vi "STED Control V6.vi"() -> ()   [LabVIEW 2014]
uses:
  FPGA-7842R-Reference.ctl
  Scan Parameters.ctl
  Manual Controls V2.ctl
  <vilib>/Utility/miscctls.llb/LVRectTypeDef.ctl
  Laser Controls.ctl
  Controls/StageStates.ctl
  <vilib>/Utility/miscctls.llb/LVPositionTypeDef.ctl
  Type Defs/Image Acquisition Parameters.ctl
  Detectors.ctl
  Type Defs/P541.ctl
  Tools VIs/GrpahTools.ctl
  Type Defs/N664.ctl
  Type Defs/M227.ctl
  Type Defs/P612.ctl
  Type Defs/M686.ctl
  Type Defs/P841.ctl
  Type Defs/ASI.ctl
  Type Defs/Image Control.ctl
panel:
  in  "Load Positions":bool
  in  "ASI":bool
  in  "4Pi Cavity Translation Z - ASI":T1={"Up ASI"=FALSE, "Down ASI"=FALSE, "Step Size (um)"=0.001, "Z (um)"=0.001, "F (um)"=0.001, "Velocity"=0.001} caption="ASI" {"Velocity" min=0.001; "F (um)" min=0.001; "Z (um)" min=0.001; "Step Size (um)" min=0.001}
  in  "Lower Shutter":bool
  in  "Upper Shutter":bool
  in  "Phase Compensation Mirror - P841 (0~15 um)":T2
  in  "Sample Stage XY - M686":T3 {"Y" format="%#_4g"; "X" format="%#_4g"}
  in  "Joystick Velocity":string(combo)
  in  "Radio Buttons":enum32{"Radio Selection 1", "Radio Selection 2"}(radio)
  in  "Bottom Objective Holder XY - P612 (0~100 um)":T4 {"Y" format="%#_4g"; "X" format="%#_4g"}
  in  "Upper Objective Holder Z - N664 (8~19 mm)":T5 {"Position" min=8.0 max=20.0 scale=8.0..20.0; "Step Size (um)" min=0.001}
  in  "Abort AllStage":bool
  in  "Stages":T6={"M227"=TRUE, "N664"=TRUE, "P612"=TRUE, "M686"=TRUE, "P841"=TRUE, "ASI"=TRUE}
  in  "Micrometer Sample Stage Holder Z - M227":T7
  in  "Cursor":bool
  in  "Graph Mode":T8=enum."FullChip"
  in  "Colormap":T9(ring)
  in  "Active Channel":u16(ring) items=["Channel 1"]
  in  "Graph Tools":T10
  in  "Tab Control":T11(tab)
  in  "SLM":bool
  in  "DM":bool
  in  "Timing":bool
  in  "Focus Control":T12
  out "Channel 6":sgl[][](graph)
  out "Channel 5":sgl[][](graph)
  out "Channel 4":sgl[][](graph)
  out "Channel 3":sgl[][](graph)
  out "Channel 2":sgl[][](graph)
  in  "Detectors":T13
  in  "Laser Controls":T14 {"STED Power (V)" scale=0.0..10.0}
  in  "Save File Path":path=path "C:/Users/ED STED/Desktop/temp.DBL"
  in  "Capture":bool
  out "Channel 1":sgl[][](graph)
  in  "Image Acquisition Parameters":T15={"Scan Type"=enum."Beam Scanning", "Scan Mode"=enum."XY", "Fast Axis Frequency (Hz)"=15780.0, "Image Format"=256, "Line Accumulations"=100, "Frames Per Capture"=1, "Frames Accumulations"=1, "Image Dimension (um)"=[15.0, 15.0], "Number of Z Steps"=1, "Z Steps Size (um)"=1.0, "Pixel Size (nm)"=[58.59375, 58.59375]} {"Z Steps Size (um)" min=0.0; "Number of Z Steps" min=1; "Frames Accumulations" min=1; "Frames Per Capture" min=1; "Line Accumulations" min=1; "Image Format" items=["64 x 64"=64, "128 x 128"=128, "256 x 256"=256, "512 x 512"=512, "1024 x 1024"=1024, "2048 x 2048"=2048]}
  in  "Live":bool
  in  "Exit":bool
  # "Sample Stage XY - M686 (0~25 mm)"
  # "XY"
  # "Z"
  # "Length"
  # "Height"
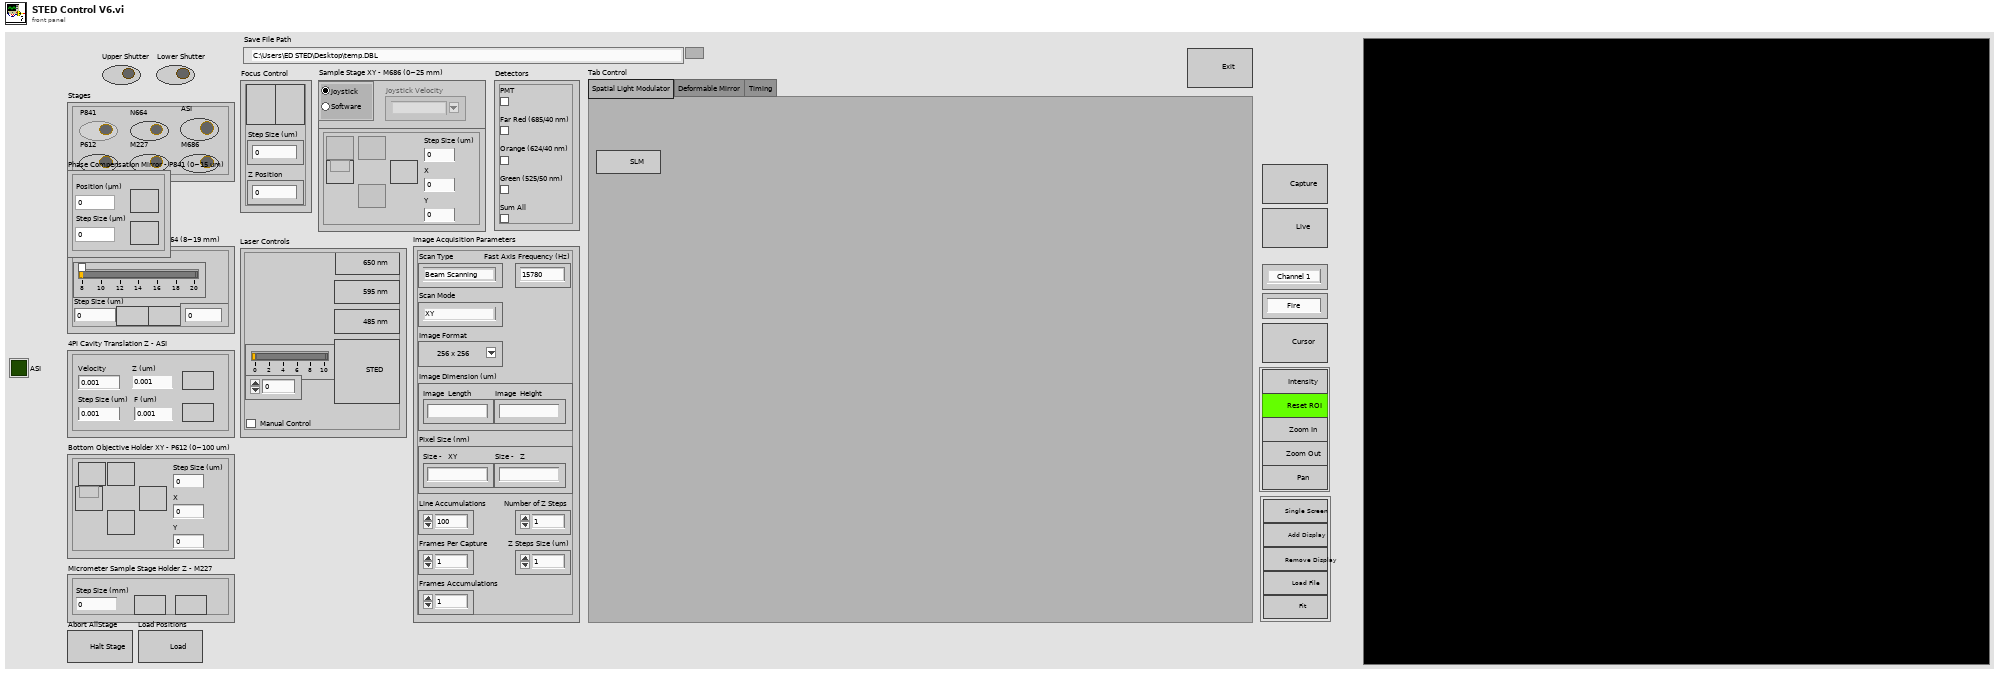
[diagram p1: front panel]
types:
  T1 = typedef "ASI.ctl" = cluster{"Up ASI":bool, "Down ASI":bool, "Step Size (um)":dbl, "Z (um)":dbl, "F (um)":dbl, "Velocity":dbl}
  T2 = typedef "P841.ctl" = cluster{"Position (µm)":dbl, "Step Size (µm)":dbl, "Up P841":bool, "Down P841":bool}
  T3 = typedef "M686.ctl" = cluster{"Home Button":bool, "Up Button":bool, "Left Button":bool, "Down Button":bool, "Right Button":bool, "Step Size (um)":dbl, "X":dbl, "Y":dbl}
  T4 = typedef "P612.ctl" = cluster{"Home Button":bool, "Up Button":bool, "Left Button":bool, "Down Button":bool, "Right Button":bool, "Step Size (um)":dbl, "X":dbl, "Y":dbl}
  T5 = typedef "N664.ctl" = cluster{"Up_N664":bool, "Down_N664":bool, "Step Size (um)":dbl, "Position":dbl}
  T6 = cluster{"M227":bool, "N664":bool, "P612":bool, "M686":bool, "P841":bool, "ASI":bool}
  T7 = typedef "M227.ctl" = cluster{"Up M227":bool, "Down M227":bool, "Step Size (mm)":dbl}
  T8 = typedef "Image Control.ctl" = enum32{"GetIntensity", "FullChip", "ZoomIn", "ZoomOut", "Pan"}
  T9 = enum16{"Fire", "Gray", "Red", "Green", "Blue", "Cyan", "Magenta", "Yellow", "Red-White", "Green-White", "Blue-White", "Glow"}
  T10 = typedef "GrpahTools.ctl" = cluster{"Add Display":bool, "Remove Display":bool, "Single Screen":bool, "Load File":bool, "Fit":bool}
  T11 = enum32{"Spatial Light Modulator", "Deformable Mirror", "Timing"}
  T12 = typedef "P541.ctl" = cluster{"Step Up":bool, "Step Down":bool, "Z Position":dbl, "Step Size (um)":dbl}
  T13 = typedef "Detectors.ctl" = cluster{"PMT":bool, "Far Red (685/40 nm)":bool, "Orange (624/40 nm)":bool, "Green (525/50 nm)":bool, "Sum All":bool}
  T14 = typedef "Laser Controls.ctl" = cluster{"STED Power (V)":dbl, "STED":bool, "640 nm":bool, "590 nm":bool, "485 nm":bool, "Manual Control":bool}
  T15 = typedef "Image Acquisition Parameters.ctl" = cluster{"Scan Type":enum16{"Sample Scanning", "Beam Scanning"}, "Scan Mode":enum16{"XY", "XZ", "YZ", "XYZ"}, "Fast Axis Frequency (Hz)":dbl, "Image Format":u16, "Line Accumulations":u16, "Frames Per Capture":u16, "Frames Accumulations":u16, "Image Dimension (um)":dbl[], "Number of Z Steps":u8, "Z Steps Size (um)":dbl, "Pixel Size (nm)":dbl[]}
  T16 = typedef "FPGA-7842R-Reference.ctl" = enum16{"Stage Control", "Laser Control", "Unused Axis I16", "Exit", "Set Res Mirror", "Set Galvo", "Default", "Close FPGA", "Stop Waveforms", "Start Waveforms", "Shutter Control", "Initialize"}
  T17 = typedef "Scan Parameters.ctl" = cluster{"Fast_Ax_Amp_V":dbl, "Fast_Ax_Off_V":dbl, "Slow_Ax_Amp_V":dbl, "Slow_Ax_Off_V ":dbl, "Slow_Ax_Max_V_VperS":dbl, "Slow_Ax1_Del25ns":i32, "Slow_Ax2_Del25ns":i32, "Stage_X_Off_V":dbl, "Stage_Y_Off_V":dbl, "Stage_Z_Off_V":dbl, "Galvo1_Off_V":dbl, "Galvo2_Off_V":dbl, "Last_Scan_Mode":enum16{"XY", "XZ", "YZ", "XYZ"}, "Current_Scan_Mode":enum16{"XY", "XZ", "YZ", "XYZ"}, "Fly_Back_Lines":u16, "Linear_Ramp_End":u32, "Z_Step_I16":i16, "Z_Start_I16":i16, "Laser_States _U32":u32, "590_Voltage_I16":i16, "775_AOM_Volt_I16":i16, "Blanking OFF":bool, "Unused_Axis_I16":i16}
  T18 = typedef "Manual Controls V2.ctl" = cluster{"Galvo 1 Position (I16)":i16, "Galvo 2 Position (I16)":i16, "X Axis Voltage (I16)":i16, "Y Axis Voltage (I16)":i16, "Z Axis Voltage (I16)":i16, "Res Mirror Amp (I16)":i16, "Res Mirror Mute":bool, "Upper Shutter":bool, "Lower Shutter":bool}
  T19 = enum8{"Enabled", "Disabled", "Disabled and Grayed Out"}
  T20 = typedef "LVPositionTypeDef.ctl" = cluster{"Left":i32, "Top":i32}
  T21 = typedef "LVRectTypeDef.ctl" = cluster{"Left":i16, "Top":i16, "Right":i16, "Bottom":i16}
  T22 = enum32{"Invalid", "Standard", "Closed", "Hidden", "Minimized", "Maximized"}
  T23 = typedef "StageStates.ctl" = enum16{"POSITION", "MVR", "MOVE", "HALT", "ONTARGET", "ERROR", "EXIT", "HOME", "ZEROPOS", "NANOPOS", "QUIT", "ANALOG"}
  T24 = enum16{"open", "open or create", "create or replace", "create", "open (read-only)"}
  T25 = cluster{"Down_N664":bool, "Down_N664":bool, "Step Size (um)":dbl, "Numeric":dbl}
  T26 = cluster{bool, bool, bool, bool, bool, dbl, "Numeric":dbl, "Numeric":dbl}
  T27 = cluster{bool, bool, dbl, dbl, "Numeric":dbl, "Numeric":dbl, dbl}
  T28 = cluster{"Scan Type":bool, "Scan Mode":bool, "Fast Axis Frequency (Hz)":bool, "Image Format":bool, "Line Accumulations":bool, "Frames Per Capture":bool, "Frames Accumulations":bool, "Image Dimension (um)":bool[], "Number of Z Steps":bool, "Z Steps Size (um)":bool, "Pixel Size (nm)":bool[]}
  T29 = typedef "LVAllMonitorsDisplayTypeDef.ctl" = cluster{"Bounds":cluster{"Left":i16, "Top":i16, "Right":i16, "Bottom":i16}, "Depth":i16}[]
  T30 = cluster{"Bounds":cluster{"Left":i16, "Top":i16, "Right":i16, "Bottom":i16}, "Depth":i16}
  T31 = cluster{bool, bool, bool, bool, bool, "Step Size (um)":dbl, "Numeric":dbl, "Numeric":dbl}
  T32 = cluster{bool, bool, "Step Size (um)":dbl, dbl, "Numeric":dbl, "Numeric":dbl, "Velocity":dbl}
  T33 = cluster{"Upper Shutter":bool, "Upper Shutter":bool}
  T34 = enum32{"GetIntensity", "FullChip", "ZoomIn", "ZoomOut", "Pan"}
  T35 = typedef "IMAQ Image.ctl" = refnum<image>
  T36 = typedef "Waveform Data.ctl" = cluster{"Waveform Scan Parameters":cluster{"Scanning Mode":u8, "Fast Axis WF Length (Elements)":i32, "Fast Axis Sample Period (Ticks)":u32, "Slow Axis 1 WF Length (Elements)":i32, "Slow Axis 1 Sample Period (Ticks)":u32, "Slow Axis 1 Delay (25 ns) Steps":i32, "Slow Axis 2 WFLength (Elements)":i32, "Slow Axis 2 Sample Period (Ticks)":u32, "Slow Axis 2 Delay (25 ns) Steps":i32}, "Fast Axis Waveform":dbl[], "Slow Axis 1 Waveform":dbl[], "Slow Axis 2 Waveform":dbl[]}
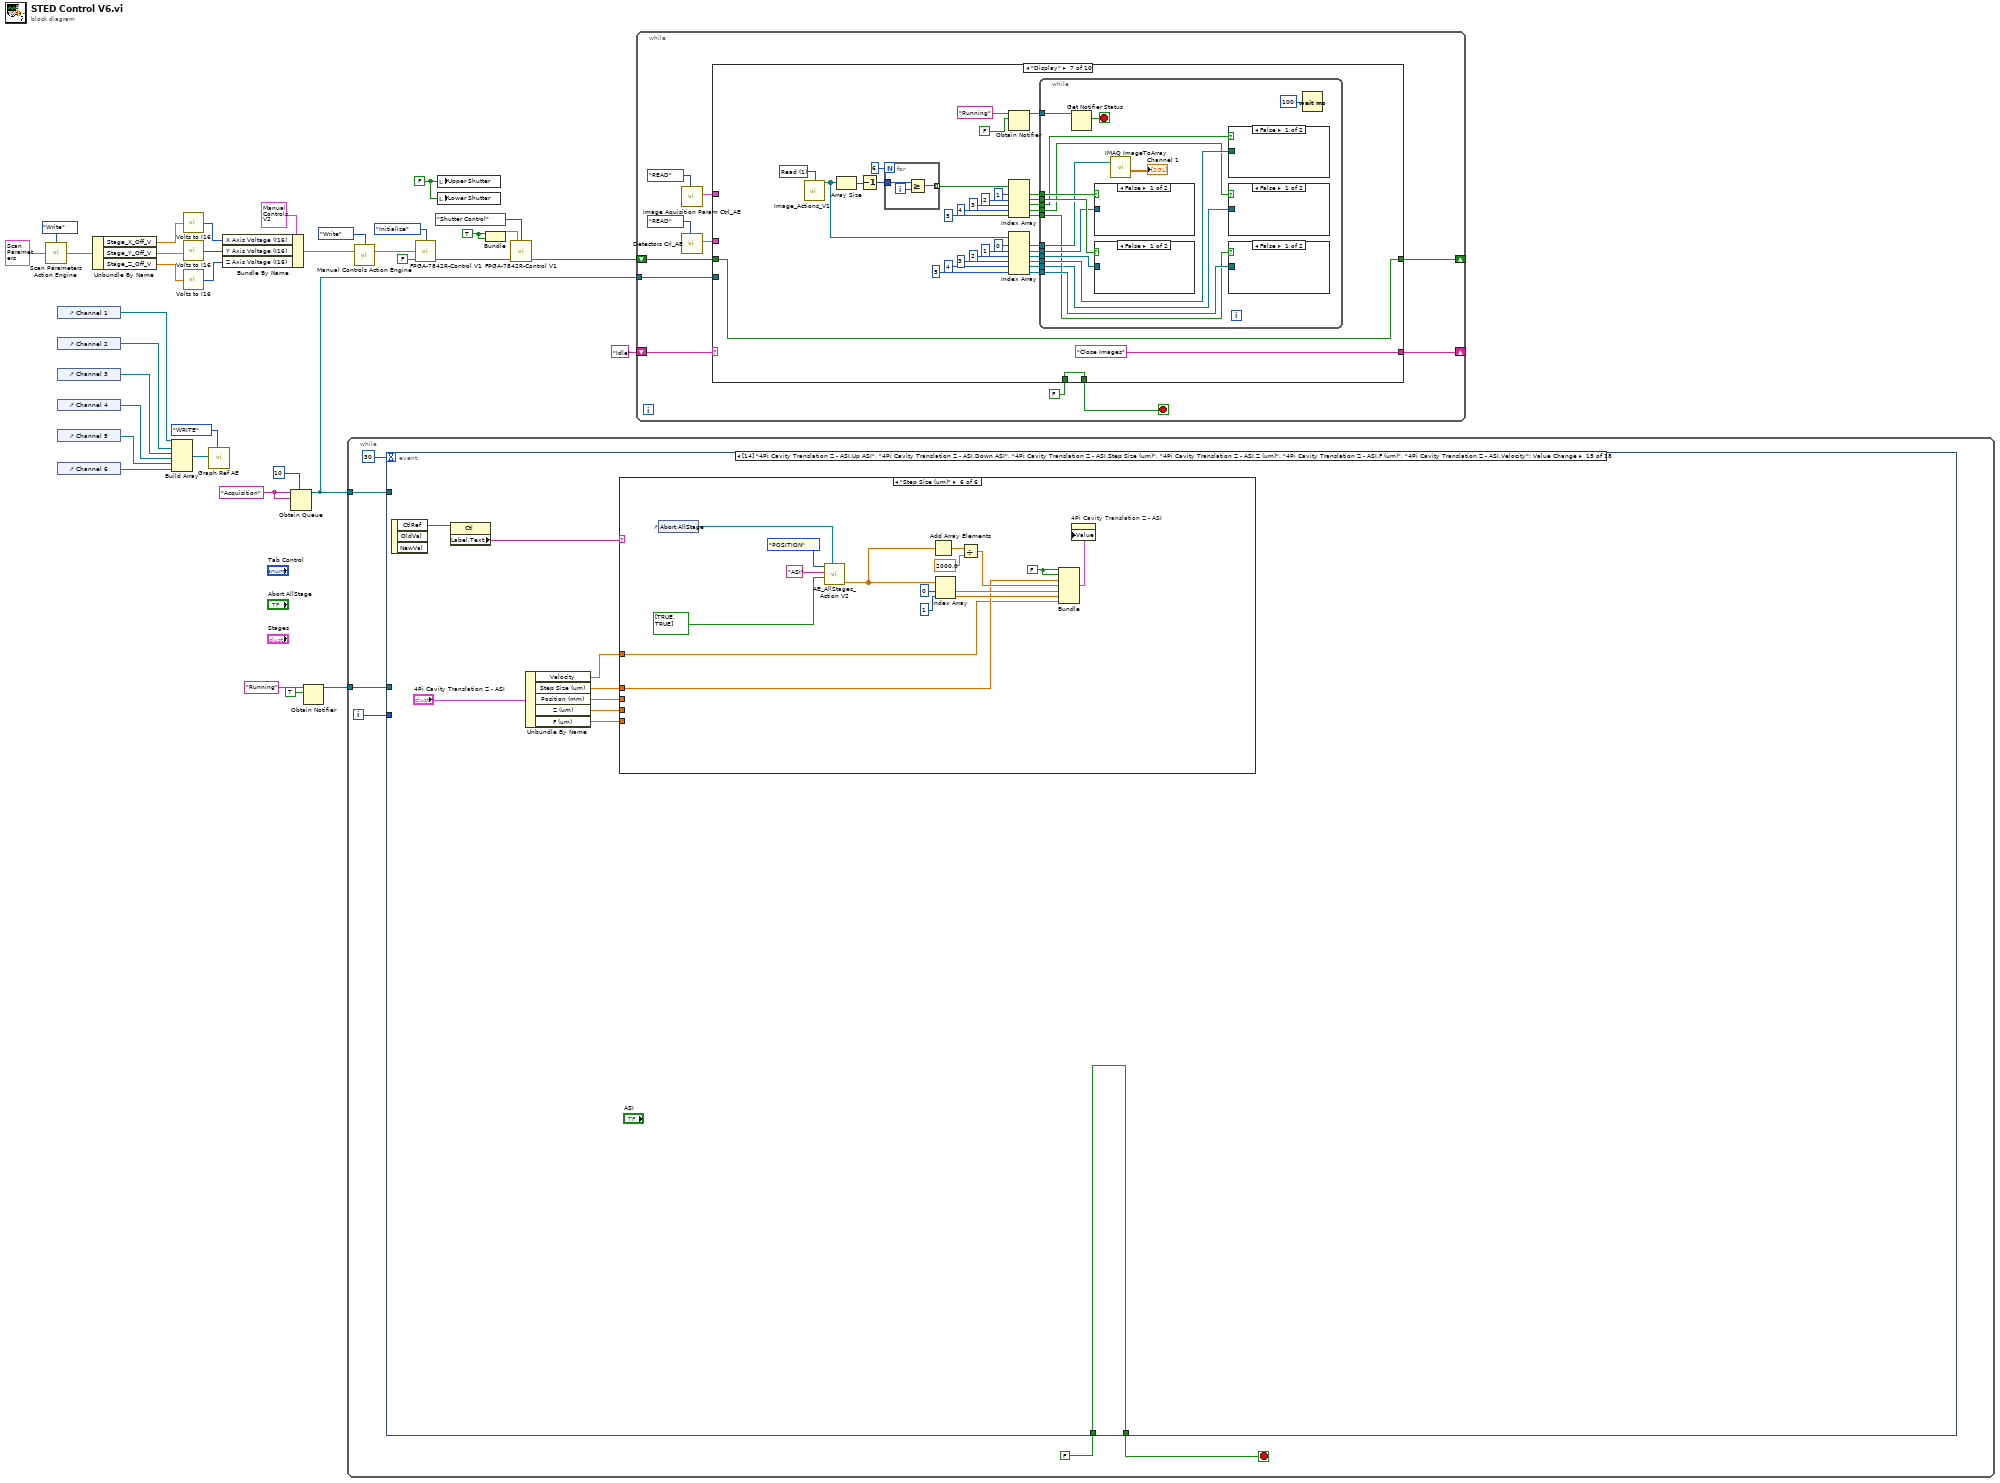
[diagram p0: block diagram]
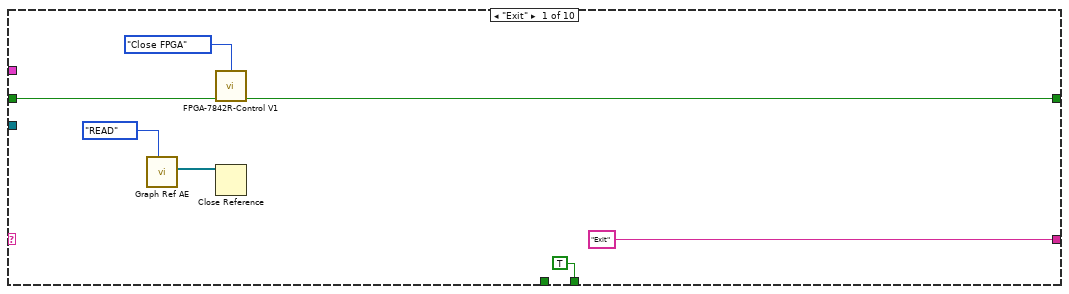
[diagram p2: hidden frame]
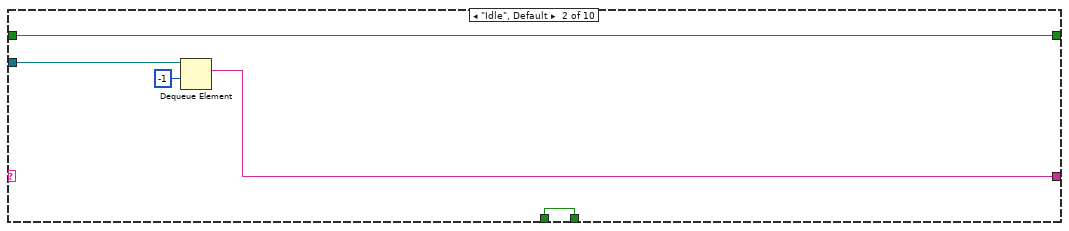
[diagram p3: hidden frame]
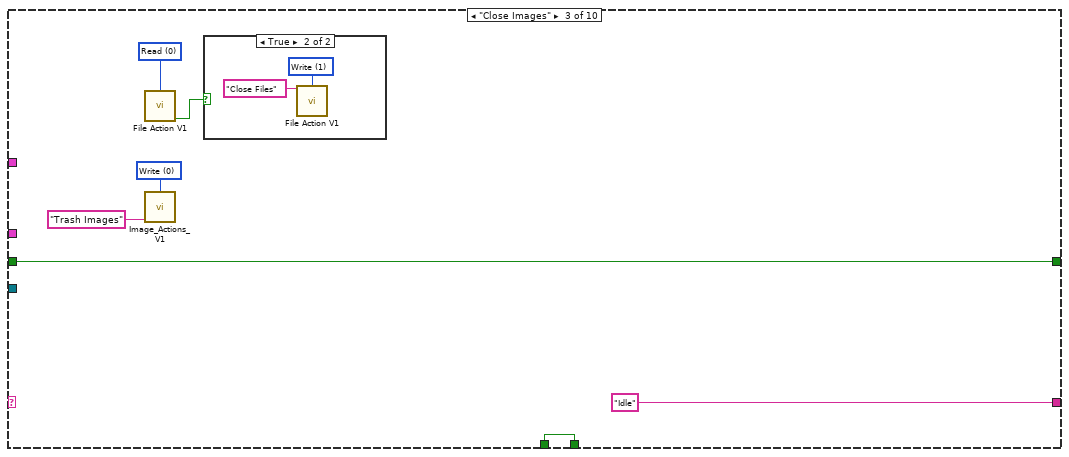
[diagram p4: hidden frame]
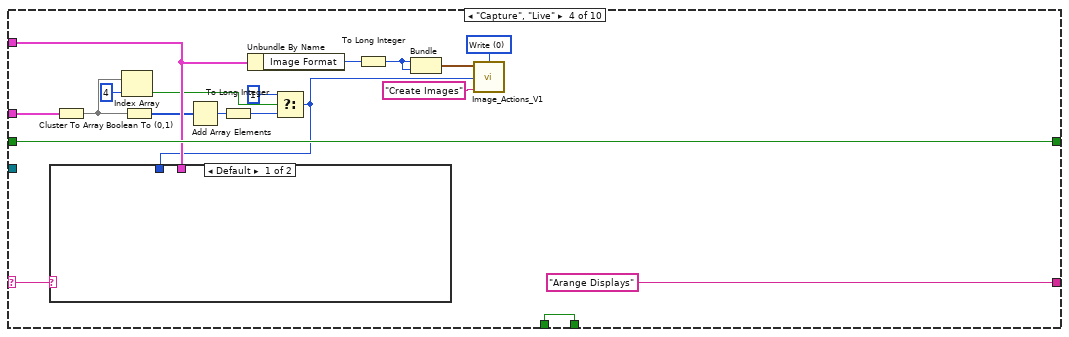
[diagram p6: hidden frame]
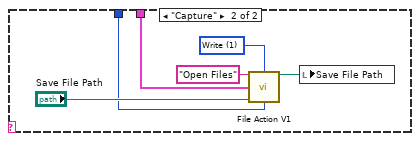
[diagram p7: hidden frame]
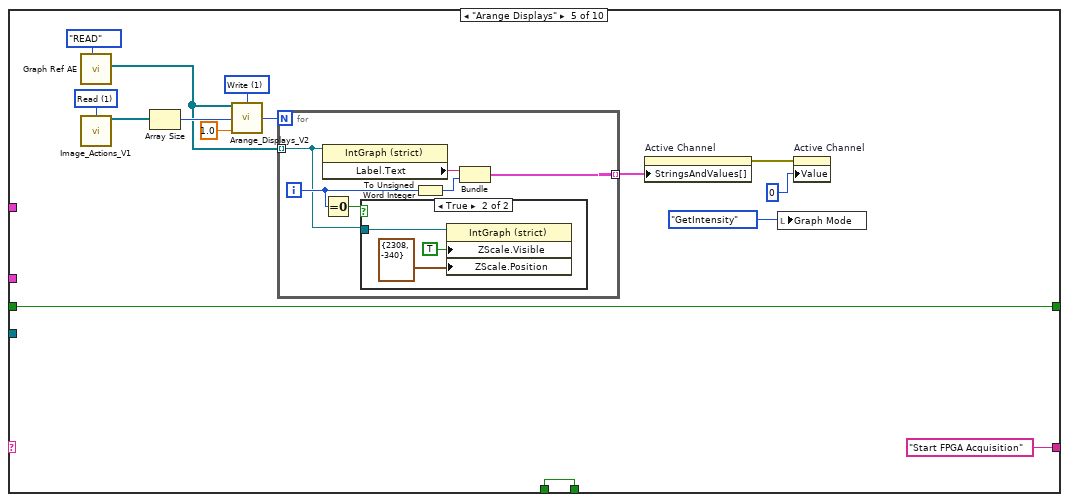
[diagram p8: hidden frame]
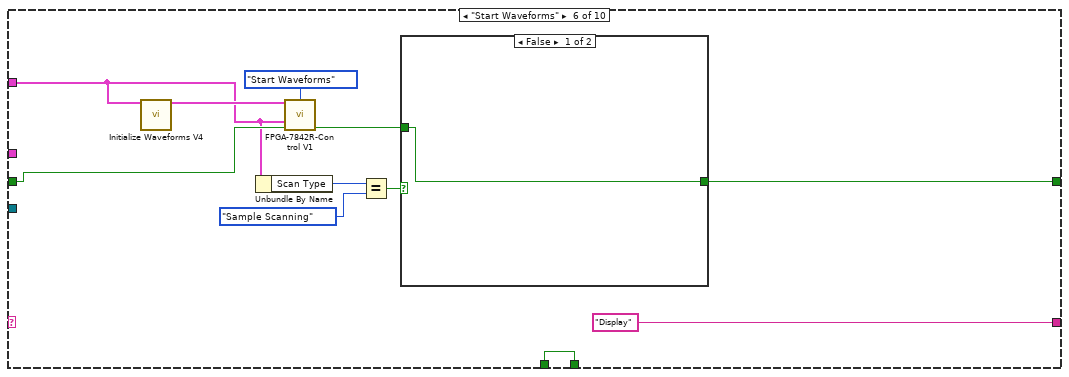
[diagram p10: hidden frame]
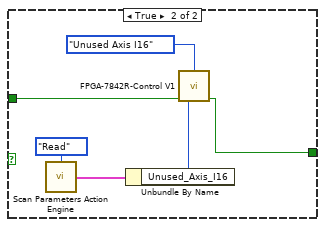
[diagram p11: hidden frame]
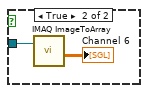
[diagram p12: hidden frame]
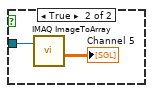
[diagram p13: hidden frame]
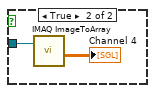
[diagram p14: hidden frame]
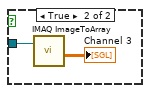
[diagram p15: hidden frame]
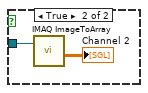
[diagram p16: hidden frame]
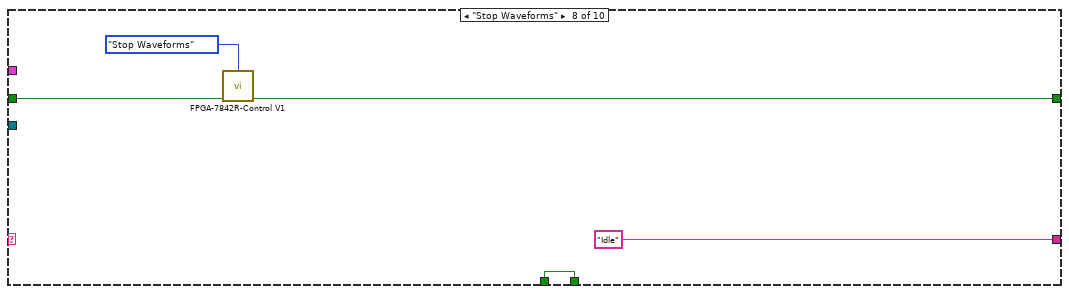
[diagram p17: hidden frame]
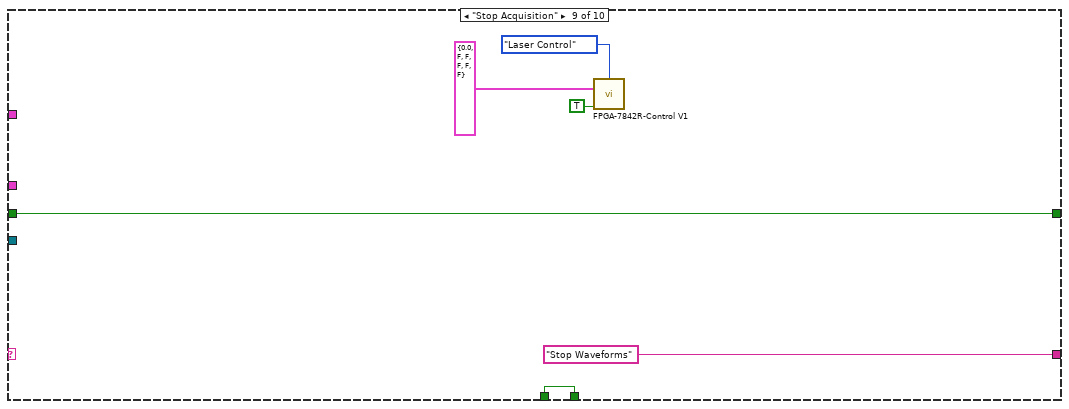
[diagram p18: hidden frame]
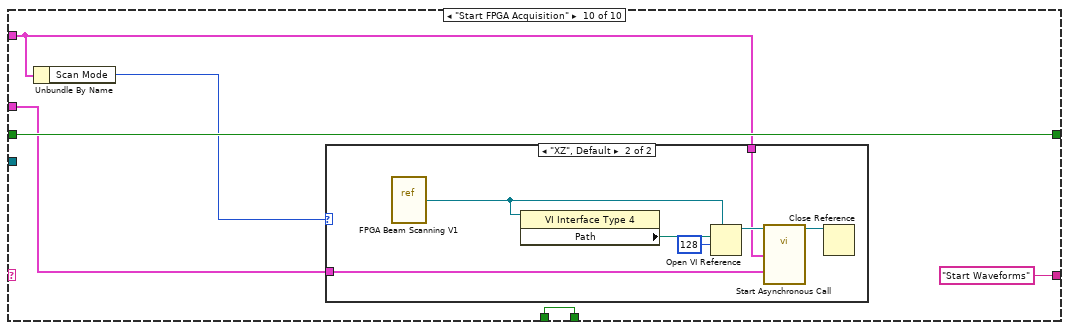
[diagram p19: hidden frame]
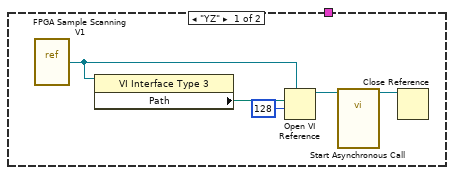
[diagram p20: hidden frame]
diagram:
  w2 = TRUE ("Upper Shutter")
  w10 = "Acquisition" ("name (unnamed)")
  w13 = FALSE ("Upper Shutter")
  n1 = call "Scan Parameters Action Engine.vi"("Action"=enum16{"Read", "Write"}."Write", "Scan Parameters IN"=T17 {"Fast_Ax_Amp_V"=0.0, "Fast_Ax_Off_V"=0.0, "Slow_Ax_Amp_V"=0.0, "Slow_Ax_Off_V "=0.0, "Slow_Ax_Max_V_VperS"=0.0, "Slow_Ax1_Del25ns"=0, "Slow_Ax2_Del25ns"=0, "Stage_X_Off_V"=5.0, "Stage_Y_Off_V"=5.0, "Stage_Z_Off_V"=5.0, "Galvo1_Off_V"=0.0, "Galvo2_Off_V"=0.0, "Last_Scan_Mode"=enum."XY", "Current_Scan_Mode"=enum."XY", "Fly_Back_Lines"=0, "Linear_Ramp_End"=0, "Z_Step_I16"=0, "Z_Start_I16"=0, "Laser_States _U32"=0, "590_Voltage_I16"=0, "775_AOM_Volt_I16"=0, "Blanking OFF"=FALSE, "Unused_Axis_I16"=16384}) -> ("Scan Parameters OUT"=w24:T17)  [unwired: 13 in]
  n2 = control-ref of="Channel 1"() -> (w16:refnum<vi>)
  n3 = control-ref of="Channel 2"() -> (w32:refnum<vi>)
  n4 = control-ref of="Channel 3"() -> (w17:refnum<vi>)
  n5 = control-ref of="Channel 4"() -> (w31:refnum<vi>)
  n6 = control-ref of="Channel 5"() -> (w30:refnum<vi>)
  n7 = control-ref of="Channel 6"() -> (w29:refnum<vi>)
  n8 = Unbundle By Name(w24) -> ("Stage_X_Off_V"=w20:dbl, "Stage_Y_Off_V"=w19:dbl, "Stage_Z_Off_V"=w18:dbl)
  n9 = Build Array(w16, w32, w17, w31, w30, w29) -> (w14:refnum<vi>[])
  n10 = call "Volts to I16.vi"("Voltage (V)"=w20) -> ("I16"=w21:i16)  [unwired: 13 in, 1 out]
  n11 = call "Volts to I16.vi"("Voltage (V)"=w19) -> ("I16"=w22:i16)  [unwired: 13 in, 1 out]
  n12 = call "Volts to I16.vi"("Voltage (V)"=w18) -> ("I16"=w23:i16)  [unwired: 13 in, 1 out]
  n13 = call "Graph Ref AE.vi"("Action"=enum16{"READ", "WRITE"}."WRITE", "Graph Ref In"=w14) -> ()  [unwired: 9 in, 1 out]
  n14 = Bundle By Name(cluster=T18 {"Galvo 1 Position (I16)"=-280, "Galvo 2 Position (I16)"=0, "X Axis Voltage (I16)"=16384, "Y Axis Voltage (I16)"=16384, "Z Axis Voltage (I16)"=16384, "Res Mirror Amp (I16)"=0, "Res Mirror Mute"=FALSE, "Upper Shutter"=FALSE, "Lower Shutter"=FALSE} ("Manual Controls"), "X Axis Voltage (I16)"=w21, "Y Axis Voltage (I16)"=w22, "Z Axis Voltage (I16)"=w23) -> (w25:T18)
  n15 = Obtain Queue(max queue size (-1, unlimited)=10, name (unnamed)=w10, element data type=w10) -> (queue out=w12:refnum<queue>)  [unwired: 2 in, 2 out]
  n16 = Obtain Notifier(name (unnamed)="Running", notification data type=TRUE) -> (notifier out=w6:refnum<notifier>)  [unwired: 2 in, 2 out]
  n17 = while {
    tunnel: w12 -> [w40]
    tunnel: w6 -> [w37]
    i -> [w38]
    stop <- w42 stop-if-true
    n18 = event shown="[14] \"4Pi Cavity Translation Z - ASI.Up ASI\", \"4Pi Cavity Translation Z - ASI.Down ASI\", \"4Pi Cavity Translation Z - ASI.Step Size (um)\", \"4Pi Cavity Translation Z - ASI.Z (um)\", \"4Pi Cavity Translation Z - ASI.F (um)\", \"4Pi Cavity Translation Z - ASI.Velocity\": Value Change" {
      selector: _ -> [_ _ _ _ _ _ _ _ _ _ _ _ _ _ _ _ _ _]
      dyn-events: _ -> [_ _ _ _ _ _ _ _ _ _ _ _ _ _ _ _ _ _]
      timeout: 30 -> [_ _ _ _ _ _ _ _ _ _ _ _ _ _ _ _ _ _]
      tunnel: [w51 w137 w151 w173 w209 w237 w315 w417 w468 w631 w647 w706 w897 w1127 w1147 w1343 w1359 w1464] -> w42
      tunnel: FALSE -> [w51 w137 w151 w173 w209 w237 w315 w417 w468 w631 w647 w706 w897 w1127 w1147 w1343 w1359 _]
      tunnel: w40 -> [w48 w136 _ _ _ _ _ _ _ _ _ _ _ _ _ _ _ w1463]
      tunnel: w38 -> [w46 _ _ _ _ _ _ _ _ _ _ _ _ _ _ _ _ _]
      tunnel: w37 -> [w43 w129 _ _ _ _ _ _ _ _ _ _ _ _ _ _ _ w1453]
      event Timeout {
        n19 = event-data() -> ()  [unwired: 1 in, 3 out]
        n20 = Equal To 0?(x=w46) -> (x = 0?=w45:bool)
        n21 = Get Notifier Status(notifier=w43) -> (current notification=w50:bool)  [unwired: 1 in, 4 out]
        n22 = case shown="True" w45 {
          frame False {
            n23 = call "Image Aquisition Param Ctrl_AE.vi"("Action"=enum16{"READ", "WRITE"}."READ") -> ("Image Acquisition Parameters Out"=w55:T15)  [unwired: 10 in]
            n24 = call "Detectors Crl_AE.vi"("Action"=enum16{"READ", "WRITE"}."READ") -> ("Detectors Parameters Out"=w56:T13)  [unwired: 10 in]
            n25 = call "LASERs_ Crl_AE.vi"("Action"=enum16{"READ", "WRITE"}."READ") -> ("Detectors Parameters Out"=w57:T14)  [unwired: 10 in]
            n26 = local write "Image Acquisition Parameters"(w55) -> ()
            n27 = local write "Detectors"(w56) -> ()
            n28 = local write "Laser Controls"(w57) -> ()
          }
          frame True {
            n29 = local read "Image Acquisition Parameters"() -> (w63:T15)
            n30 = local read "Laser Controls"() -> (w61:T14)
            n31 = local read "Detectors"() -> (w60:T13)
            n32 = call "Image Aquisition Param Ctrl_AE.vi"("Action"=enum16{"READ", "WRITE"}."WRITE", "Image Acquisition Parameters In"=w63) -> ()  [unwired: 9 in, 1 out]
            n33 = call "Detectors Crl_AE.vi"("Action"=enum16{"READ", "WRITE"}."WRITE", "Detectors Parameters In"=w60) -> ()  [unwired: 9 in, 1 out]
            n34 = call "LASERs_ Crl_AE.vi"("Action"=enum16{"READ", "WRITE"}."WRITE", "Detectors Parameters In"=w61) -> ()  [unwired: 9 in, 1 out]
            n35 = property on="Stages" class="Clust (strict)"() -> ("Controls[]"=w58:refnum<vi>[])  [unwired: 2 in, 2 out]
            n36 = for {
              tunnel: w58 -> [w68] mode=indexing
              n37 = property class="Ctl"(reference=w68) -> ("Label.Text"=w66:string, "Value"=w70:variant)  [unwired: 1 in, 2 out]
              n38 = Variant To Data(type=TRUE, Variant=w70) -> (data=w67:bool)  [unwired: 1 in, 1 out]
              n39 = call "All_Stages_Aloha.vi"("Aloha"=w67, "Stage ID"=w66) -> ("Position Out"=w65:dbl[])  [unwired: 9 in]
              n40 = case shown="\"ASI\"" w66 {
                tunnel: w65 -> [_ _ w77 w84 w98 w108 w113]
                frame "0", Default {
                }
                frame "M227" {
                  w74 = FALSE
                  n41 = Bundle(w74, w74, 1.0) -> (w72:cluster{bool, bool, dbl})  [unwired: 1 in]
                  n42 = To Variant(anything=w72) -> (Variant=w71:variant)
                  n43 = property on="Micrometer Sample Stage Holder Z - M227" class="Clust"("Value"=w71) -> ()  [unwired: 2 in, 2 out]
                }
                frame "N664" {
                  w80 = FALSE ("Down_N664")
                  n44 = Index Array(array=w77, index=0) -> (element=w78:dbl)
                  n45 = Bundle("Down_N664"=w80, "Down_N664"=w80, "Step Size (um)"=1.0, "Numeric"=w78) -> (w76:T25)  [unwired: 1 in]
                  n46 = To Variant(anything=w76) -> (Variant=w75:variant)
                  n47 = property on="Upper Objective Holder Z - N664 (8~19 mm)" class="Clust"("Value"=w75) -> ()  [unwired: 2 in, 2 out]
                }
                frame "P612" {
                  w86 = FALSE
                  w96 = FALSE
                  n48 = Index Array(array=w84, index #1=0, index #2=1, index #3=2 ("index")) -> (element #1=w93:dbl, element #2=w91:dbl, element #3=w87:dbl)
                  n49 = Bundle(w96, w96, w96, w96, w96, 1.0, "Numeric"=w93, "Numeric"=w91) -> (w92:T26)  [unwired: 1 in]
                  n50 = Bundle(w86, w86, i16 0, w86, "Numeric"=w87) -> (w88:cluster{bool, bool, i16, bool, "Numeric":dbl})  [unwired: 1 in]
                  n51 = To Variant(anything=w92) -> (Variant=w83:variant)
                  n52 = To Variant(anything=w88) -> (Variant=w82:variant)
                  n53 = property on="Bottom Objective Holder XY - P612 (0~100 um)" class="Clust"("Value"=w83) -> ()  [unwired: 2 in, 2 out]
                  n54 = property on="Focus Control" class="Clust"("Value"=w82) -> ()  [unwired: 2 in, 2 out]
                }
                frame "M686" {
                  w107 = FALSE
                  n55 = Index Array(array=w98, index #1=0, index #2=1) -> (element #1=w104:dbl, element #2=w99:dbl)
                  n56 = Bundle(w107, w107, w107, w107, w107, 10.0, "Numeric"=w104, "Numeric"=w99) -> (w103:T26)  [unwired: 1 in]
                  n57 = To Variant(anything=w103) -> (Variant=w97:variant)
                  n58 = property on="Joystick Velocity" class="CmbBox"("DisabledEnum"=T19."Disabled and Grayed Out" ("Disabled")) -> ()  [unwired: 2 in, 2 out]
                  n59 = property on="Radio Buttons" class="RadioBtnsControl (strict)"("Value"=enum32{"Radio Selection 1", "Radio Selection 2"}."Radio Selection 2" ("Radio Buttons")) -> ()  [unwired: 2 in, 2 out]
                  n60 = property on="Sample Stage XY - M686" class="Clust"("Value"=w97) -> ()  [unwired: 2 in, 2 out]
                }
                frame "P841" {
                  n61 = Index Array(array=w108, index=0) -> (element=w110:dbl)
                  n62 = Bundle("Numeric"=w110) -> (w109:cluster{"Numeric":dbl})  [unwired: 1 in]
                  n63 = property on="Phase Compensation Mirror - P841 (0~15 um)" class="Clust"("Value"=w109) -> ()  [unwired: 2 in, 2 out]
                }
                frame "ASI" {
                  w116 = FALSE
                  n64 = Add Array Elements(numeric array=w113) -> (sum=w120:dbl)
                  n65 = Index Array(array=w113, index #1=0 ("index"), index #2=1 ("index")) -> (element #1=w122:dbl, element #2=w121:dbl)
                  n66 = Divide(x=w120, y=2000.0) -> (x/y=w118:dbl)
                  n67 = Bundle(w116, w116, 1.0, w118, "Numeric"=w122, "Numeric"=w121, 1.0) -> (w115:T27)  [unwired: 1 in]
                  n68 = To Variant(anything=w115) -> (Variant=w112:variant)
                  n69 = property on="4Pi Cavity Translation Z - ASI" class="Clust"("Value"=w112) -> ()  [unwired: 2 in, 2 out]
                }
              }
            }
          }
        }
        n70 = local read "Capture"() -> (w49:bool)
        n71 = And(x=w50, y=w49) -> (x .and. y?=w47:bool)
        n72 = local write "ASI"(FALSE ("Moving")) -> ()
        n73 = case shown="True" w47 {
          tunnel: w48 -> [_ w127]
          frame False {
          }
          frame True {
            n74 = local write "Capture"(FALSE ("Capture")) -> ()
            n75 = Enqueue Element(queue=w127, element="Stop Acquisition" ("f")) -> ()  [unwired: 2 in, 3 out]
            n76 = property on="Live" class="Bool (strict)"("DisabledEnum"=T19."Enabled" ("Disabled")) -> ()  [unwired: 2 in, 2 out]
          }
        }
      }
      event "Live", "Capture": Value Change {
        n77 = event-data() -> ("CtlRef"=w135:refnum<vi>, "NewVal"=w130:bool)  [unwired: 1 in]
        n78 = Not(x=w130) -> (.not. x?=w133:bool)
        n79 = property class="Bool (strict)"(reference=w135) -> ("Label.Text"=w131:string)  [unwired: 1 in, 2 out]
        n80 = Send Notification(notification=w133, notifier=w129) -> ()  [unwired: 1 in, 2 out]
        n81 = case shown="\"Capture\"" w131 {
          tunnel: w130 -> [_ w139 w143]
          frame "False", Default {
          }
          frame "Live" {
            n82 = case shown="True" w139 {
              tunnel: [T19."Enabled" ("Disabled") T19."Disabled and Grayed Out" ("Disabled")] -> w138
              frame False {
              }
              frame True {
              }
            }
            n83 = property on="Capture" class="Bool (strict)"("DisabledEnum"=w138) -> ()  [unwired: 2 in, 2 out]
            n84 = property on="Exit" class="Bool"("DisabledEnum"=w138) -> ()  [unwired: 2 in, 2 out]
          }
          frame "Capture" {
            n85 = case shown="True" w143 {
              tunnel: [T19."Enabled" ("Disabled") T19."Disabled and Grayed Out" ("Disabled")] -> w142
              frame False {
              }
              frame True {
              }
            }
            n86 = property on="Live" class="Bool (strict)"("DisabledEnum"=w142) -> ()  [unwired: 2 in, 2 out]
            n87 = property on="Exit" class="Bool"("DisabledEnum"=w142) -> ()  [unwired: 2 in, 2 out]
          }
        }
        n88 = Select(t=w131, s=w130, f="Stop Acquisition") -> (s? t:f=w132:string)
        n89 = Enqueue Element(queue=w136, element=w132) -> ()  [unwired: 2 in, 3 out]
      }
      event Value Change {
        w159 = FALSE ("element")
        n90 = event-data() -> ()  [unwired: 1 in, 6 out]
        n91 = Unbundle By Name("Laser Controls") -> ("STED"=w165:bool, "640 nm"=w162:bool, "590 nm"=w163:bool, "485 nm"=w164:bool, "STED Power (V)"=w156:dbl, "Manual Control"=w149:bool)
        n92 = local read "Live"() -> (w150:bool)
        n93 = call "LASERs_ Crl_AE.vi"("Action"=enum16{"READ", "WRITE"}."WRITE", "Detectors Parameters In"="Laser Controls") -> ()  [unwired: 9 in, 1 out]
        n94 = Or(x=w150, y=w149) -> (x .or. y?=w148:bool)
        n95 = In Range and Coerce(upper limit=10.0, x=w156, lower limit=0.0) -> (coerced(x)=w153:dbl)  [unwired: 1 out]
        n96 = Build Array(w165, w162, w163, w164, w159, w159, w159, w159) -> (w161:bool[])
        n97 = case shown="True" w148 {
          tunnel: "Laser Controls" -> [_ w171]
          frame False {
          }
          frame True {
            n98 = call "FPGA-7842R-Control V1.vi"("Action"=FPGA-7842R-Reference."Laser Control", "Laser Controls"=w171, "Initialize"=TRUE) -> ()  [unwired: 11 in, 2 out]
          }
        }
        n99 = Boolean Array To Number(Boolean array=w161) -> (number=w160:u32)
        n100 = To Unsigned Byte Integer(number=w160) -> (unsigned 8bit integer=w158:u8)
        n101 = call "U8_To_U32.vi"("U8 IN"=w158) -> ("U32 OUT"=w157:u32)  [unwired: 13 in, 1 out]
        n102 = call "Volts to I16.vi"("Voltage (V)"=w153) -> ("I16"=w152:i16)  [unwired: 13 in, 1 out]
        n103 = call "Scan Parameters Action Engine.vi"("Action"=enum16{"Read", "Write"}."Read") -> ("Scan Parameters OUT"=w168:T17)  [unwired: 14 in]
        n104 = Bundle By Name(cluster=w168, "Laser_States _U32"=w157, "775_AOM_Volt_I16"=w152) -> (w166:T17)
        n105 = call "Scan Parameters Action Engine.vi"("Action"=enum16{"Read", "Write"}."Write", "Scan Parameters IN"=w166) -> ()  [unwired: 13 in, 1 out]
      }
      event Value Change {
        n106 = event-data() -> ()  [unwired: 1 in, 6 out]
        n107 = call "Detectors Crl_AE.vi"("Action"=enum16{"READ", "WRITE"}."WRITE", "Detectors Parameters In"="Detectors") -> ()  [unwired: 9 in, 1 out]
      }
      event Value Change {
        n108 = event-data() -> ("NewVal"=w177:T15, "OldVal"=w193:T15)  [unwired: 1 in]
        n109 = Not Equal?(x=w177, y=w193) -> (x != y?=w198:T28)
        n110 = Unbundle By Name(w198) -> ("Image Dimension (um)"=w180:bool[], "Image Format"=w178:bool, "Pixel Size (nm)"=w179:bool[])
        n111 = Or Array Elements(Boolean array=w180) -> (logical OR=w184:bool)
        n112 = Or Array Elements(Boolean array=w179) -> (logical OR=w183:bool)
        n113 = Build Array(w184, w178, w183) -> (w182:bool[])
        n114 = Boolean Array To Number(Boolean array=w182) -> (number=w181:u32)
        n115 = case shown="1, 2" w181 {
          tunnel: w180 -> [_ w221 _]
          tunnel: w177 -> [w210 w214 w228]
          tunnel: [w210 w211 w225] -> w176
          tunnel: w179 -> [_ _ w224]
          frame 0, Default {
          }
          frame 1, 2 {
            # "Image Dimension or Format Change"
            n116 = Unbundle By Name(w214) -> ("Image Dimension (um)"=w220:dbl[], "Image Format"=w218:u16)
            n117 = for {
              tunnel: w221 -> [w223] mode=indexing
              tunnel: w220 -> [w222] mode=indexing
              tunnel: [w222] -> w219
              stop <- w223 stop-if-true
            }
            n118 = To Double Precision Float(number=w218) -> (double precision float=w217:dbl)
            n119 = Build Array(w219, w219) -> (w212:dbl[])
            n120 = Divide(x=w212, y=w217) -> (x/y=w216:dbl[])
            n121 = Multiply(x=w216, y=1000.0) -> (x*y=w213:dbl[])
            n122 = Bundle By Name(cluster=w214, "Image Dimension (um)"=w212, "Pixel Size (nm)"=w213) -> (w211:T15)
          }
          frame 4 {
            # "Pixel Size Change"
            n123 = Unbundle By Name(w228) -> ("Pixel Size (nm)"=w234:dbl[], "Image Format"=w232:u16)
            n124 = for {
              tunnel: w224 -> [w236] mode=indexing
              tunnel: w234 -> [w235] mode=indexing
              tunnel: [w235] -> w233
              stop <- w236 stop-if-true
            }
            n125 = Build Array(w233, w233) -> (w226:dbl[])
            n126 = To Double Precision Float(number=w232) -> (double precision float=w231:dbl)
            n127 = Multiply(x=w226, y=w231) -> (x*y=w230:dbl[])
            n128 = Multiply(x=w230, y=0.001) -> (x*y=w227:dbl[])
            n129 = Bundle By Name(cluster=w228, "Pixel Size (nm)"=w226, "Image Dimension (um)"=w227) -> (w225:T15)
          }
        }
        n130 = Unbundle By Name(w176) -> ("Image Dimension (um)"=w199:dbl[], "Scan Mode"=w187:enum16{"XY", "XZ", "YZ", "XYZ"})
        n131 = Not Equal?(x=w187, y=enum16{"XY", "XZ", "YZ", "XYZ"}."YZ") -> (x != y?=w185:bool)
        n132 = Index Array(array=w199, index=0) -> (element=w204:dbl)
        n133 = Select(t=15780.0, s=w185, f=200.0) -> (s? t:f=w190:dbl)
        n134 = call "Res Mirror um to Volts.vi"("Image Size (um)"=w204) -> ("Voltage (V)"=w205:dbl)
        n135 = Bundle By Name(cluster=w176, "Fast Axis Frequency (Hz)"=w190) -> (w189:T15)
        n136 = In Range and Coerce(upper limit=5.0, x=w205, lower limit=0.0) -> (coerced(x)=w206:dbl)  [unwired: 1 out]
        n137 = call "Volts to I16.vi"("Voltage (V)"=w206) -> ("I16"=w203:i16)  [unwired: 13 in, 1 out]
        n138 = call "Manual Controls Action Engine.vi"("Action"=enum16{"Read", "Write"}."Read") -> ("Manual Controls Out"=w196:T18)  [unwired: 14 in]
        n139 = Bundle By Name(cluster=w196, "Res Mirror Amp (I16)"=w203, "Res Mirror Mute"=w185) -> (w194:T18)
        n140 = call "Image Aquisition Param Ctrl_AE.vi"("Action"=enum16{"READ", "WRITE"}."WRITE", "Image Acquisition Parameters In"=w189) -> ()  [unwired: 9 in, 1 out]
        n141 = call "FPGA-7842R-Control V1.vi"("Action"=FPGA-7842R-Reference."Set Res Mirror", "Manual Controls"=w194, "Initialize"=TRUE) -> ()  [unwired: 11 in, 2 out]
        n142 = call "Manual Controls Action Engine.vi"("Action"=enum16{"Read", "Write"}."Write", "Manual Controls In"=w194) -> ()  [unwired: 13 in, 1 out]
      }
      event "Active Channel", "Colormap", "Cursor": Value Change {
        n143 = event-data() -> ("CtlRef"=w240:refnum<vi>)  [unwired: 1 in, 5 out]
        n144 = property class="Ctl"(reference=w240) -> ("Label.Text"=w239:string)  [unwired: 1 in, 2 out]
        n145 = call "Graph Ref AE.vi"("Action"=enum16{"READ", "WRITE"}."READ") -> ("Graph Ref Out"=w238:refnum<vi>[])  [unwired: 10 in]
        n146 = case shown="\"Cursor\"" w239 {
          tunnel: w238 -> [w245 w277 w303 w314]
          tunnel: "Active Channel" -> [w244 w276 w302 _]
          frame "Colormap", Default {
            n147 = To Long Integer(number=w244) -> (32bit integer=w243:i32)
            n148 = Index Array(array=w245, index=w243) -> (element=w247:refnum<vi>)
            n149 = property class="IntGraph (strict)"(reference=w247) -> (reference out=w249:refnum<vi>, "ZScale.Maximum"=w248:dbl)  [unwired: 1 in, 1 out]
            n150 = case shown="\"Glow\"" "Colormap" {
              tunnel: [cluster{dbl, u32}[] [{0.0, 0}, {85.0, 16711680}, {108.0, 16729344}, {127.0, 16744192}, {132.0, 16747520}, {140.0, 16753920}, {157.0, 16766720}, {170.0, 16776960}, {245.0, 16777184}, {250.0, 16777200}, {255.0, 16777215}] ("Z Scale.Marker Values[]") cluster{dbl, u32}[] [{0.0, 0}, {255.0, 16777215}] ("Z Scale.Marker Values[]") cluster{dbl, u32}[] [{0.0, 0}, {255.0, 16711680}] ("Z Scale.Marker Values[]") cluster{dbl, u32}[] [{0.0, 0}, {255.0, 65280}] ("Z Scale.Marker Values[]") cluster{dbl, u32}[] [{0.0, 0}, {255.0, 255}] ("Z Scale.Marker Values[]") cluster{dbl, u32}[] [{0.0, 0}, {255.0, 65535}] ("Z Scale.Marker Values[]") cluster{dbl, u32}[] [{0.0, 0}, {255.0, 16711935}] ("Z Scale.Marker Values[]") cluster{dbl, u32}[] [{0.0, 0}, {255.0, 16776960}] ("Z Scale.Marker Values[]") cluster{dbl, u32}[] [{0.0, 0}, {170.0, 16711680}, {245.0, 16777184}, {250.0, 16777200}, {255.0, 16448250}] ("Z Scale.Marker Values[]") cluster{dbl, u32}[] [{0.0, 0}, {170.0, 65280}, {245.0, 16777184}, {250.0, 16777200}, {255.0, 16448250}] ("Z Scale.Marker Values[]") cluster{dbl, u32}[] [{0.0, 0}, {170.0, 255}, {245.0, 16777184}, {250.0, 16777200}, {255.0, 16448250}] ("Z Scale.Marker Values[]") cluster{dbl, u32}[] [{0.0, 0}, {1.0, 131072}, {2.0, 196608}, {3.0, 327680}, {4.0, 458752}, {5.0, 589824}, {6.0, 720896}, {7.0, 851971}, {8.0, 983043}, {9.0, 1114115}, {10.0, 1245187}, {11.0, 1376259}, {12.0, 1507331}, {13.0, 1638403}, {14.0, 1769475}, {15.0, 1769479}, {16.0, 2031623}, {17.0, 2162695}, {18.0, 2293767}, {19.0, 2424839}, {20.0, 2555911}, {21.0, 2686983}, {22.0, 2818055}, {23.0, 2949127}, {24.0, 3080203}, {25.0, 3211275}, {26.0, 3342347}, {27.0, 3473419}, {28.0, 3604491}, {29.0, 3735563}, {30.0, 3866635}, {31.0, 3867403}, {32.0, 4129547}, {33.0, 4260619}, {34.0, 4391691}, {35.0, 4522763}, {36.0, 4653839}, {37.0, 4784911}, {38.0, 4915983}, {39.0, 5178127}, {40.0, 5309199}, {41.0, 5440271}, {42.0, 5571343}, {43.0, 5702415}, {44.0, 5703439}, {45.0, 5965583}, {46.0, 6096655}, {47.0, 6227727}, {48.0, 6358799}, {49.0, 6489871}, {50.0, 6620943}, {51.0, 6752015}, {52.0, 6883087}, {53.0, 7015183}, {54.0, 7146255}, {55.0, 7277327}, {56.0, 7408399}, {57.0, 7539471}, {58.0, 7670543}, {59.0, 7801615}, {60.0, 8063759}, {61.0, 8194831}, {62.0, 8326927}, {63.0, 8457999}, {64.0, 8589075}, {65.0, 8720147}, {66.0, 8851219}, {67.0, 8982291}, {68.0, 9113363}, {69.0, 9114387}, {70.0, 9376531}, {71.0, 9507603}, {72.0, 9638675}, {73.0, 9769747}, {74.0, 9901843}, {75.0, 10032915}, {76.0, 10163987}, {77.0, 10229523}, {78.0, 10295059}, {79.0, 10427155}, {80.0, 10558227}, {81.0, 10689299}, {82.0, 10820371}, {83.0, 10886931}, {84.0, 10952467}, {85.0, 11083539}, {86.0, 11214611}, {87.0, 11215635}, {88.0, 11477779}, {89.0, 11543315}, {90.0, 11608851}, {91.0, 11740947}, {92.0, 11806483}, {93.0, 11872019}, {94.0, 12004115}, {95.0, 12135187}, {96.0, 12266259}, {97.0, 12267283}, {98.0, 12398355}, {99.0, 12529427}, {100.0, 12530451}, {101.0, 12595987}, {102.0, 12530451}, {103.0, 12793619}, {104.0, 12794131}, {105.0, 12794643}, {106.0, 13056787}, {107.0, 13057299}, {108.0, 13057811}, {109.0, 13188883}, {110.0, 13320979}, {111.0, 13386515}, {112.0, 13452563}, {113.0, 13584147}, {114.0, 13584659}, {115.0, 13585171}, {116.0, 13585683}, {117.0, 13717267}, {118.0, 13848339}, {119.0, 13849363}, {120.0, 13849875}, {121.0, 13850387}, {122.0, 13981459}, {123.0, 14113555}, {124.0, 14114067}, {125.0, 14114579}, {126.0, 14115091}, {127.0, 14246675}, {128.0, 14377747}, {129.0, 14378771}, {130.0, 14379283}, {131.0, 14379539}, {132.0, 14379795}, {133.0, 14380819}, {134.0, 14511891}, {135.0, 14643987}, {136.0, 14644503}, {137.0, 14645015}, {138.0, 14645527}, {139.0, 14646039}, {140.0, 14646551}, {141.0, 14778135}, {142.0, 14909207}, {143.0, 14910231}, {144.0, 14910747}, {145.0, 14911259}, {146.0, 14911771}, {147.0, 14912283}, {148.0, 14912797}, {149.0, 15044383}, {150.0, 15175455}, {151.0, 15175967}, {152.0, 15176479}, {153.0, 15176991}, {154.0, 15177507}, {155.0, 15178019}, {156.0, 15178531}, {157.0, 15310115}, {158.0, 15441701}, {159.0, 15441959}, {160.0, 15442215}, {161.0, 15442727}, {162.0, 15443243}, {163.0, 15443755}, {164.0, 15444269}, {165.0, 15444783}, {166.0, 15444783}, {167.0, 15576367}, {168.0, 15707953}, {169.0, 15708467}, {170.0, 15708979}, {171.0, 15708981}, {172.0, 15708983}, {173.0, 15710011}, {174.0, 15710523}, {175.0, 15711037}, {176.0, 15711039}, {177.0, 15711553}, {178.0, 15843139}, {179.0, 15974213}, {180.0, 15974215}, {181.0, 15974217}, {182.0, 15974219}, {183.0, 15975755}, {184.0, 15976271}, {185.0, 15976785}, {186.0, 15977299}, {187.0, 15977301}, {188.0, 15977815}, {189.0, 15978327}, {190.0, 15978331}, {191.0, 16109917}, {192.0, 16241503}, {193.0, 16241505}, {194.0, 16242019}, {195.0, 16242535}, {196.0, 16242537}, {197.0, 16242539}, {198.0, 16243563}, {199.0, 16243567}, {200.0, 16244081}, {201.0, 16244595}, {202.0, 16244599}, {203.0, 16244601}, {204.0, 16244603}, {205.0, 16245627}, {206.0, 16245631}, {207.0, 16245633}, {208.0, 16246147}, {209.0, 16246663}, {210.0, 16377735}, {211.0, 16508811}, {212.0, 16508815}, {213.0, 16509839}, {214.0, 16509843}, {215.0, 16509845}, {216.0, 16509847}, {217.0, 16510361}, {218.0, 16510875}, {219.0, 16510879}, {220.0, 16510881}, {221.0, 16510883}, {222.0, 16511399}, {223.0, 16511911}, {224.0, 16511915}, {225.0, 16511917}, {226.0, 16511919}, {227.0, 16511923}, {228.0, 16512437}, {229.0, 16512951}, {230.0, 16512955}, {231.0, 16512957}, {232.0, 16512959}, {233.0, 16512961}, {234.0, 16512963}, {235.0, 16512967}, {236.0, 16513481}, {237.0, 16513995}, {238.0, 16513999}, {239.0, 16514001}, {240.0, 16514003}, {241.0, 16514005}, {242.0, 16514007}, {243.0, 16514011}, {244.0, 16514013}, {245.0, 16514015}, {246.0, 16514019}, {247.0, 16514021}, {248.0, 16514023}, {249.0, 16514027}, {250.0, 16514029}, {251.0, 16514031}, {252.0, 16514035}, {253.0, 16514037}, {254.0, 16514039}, {255.0, 16514043}] ("Z Scale.Marker Values[]")] -> w251
              tunnel: [w252 w254 w256 w258 w260 w262 w264 w266 w268 w270 w272 w274] -> w250
              tunnel: w248 -> [w252 w254 w256 w258 w260 w262 w264 w266 w268 w270 w272 w274]
              frame "Fire", Default {
                # "Fire"
              }
              frame "Gray" {
                # "Grayscale"
              }
              frame "Red" {
                # "Red"
              }
              frame "Green" {
                # "Green"
              }
              frame "Blue" {
                # "Blue"
              }
              frame "Cyan" {
                # "Cyan"
              }
              frame "Magenta" {
                # "Magenta"
              }
              frame "Yellow" {
                # "Yellow"
              }
              frame "Red-White" {
                # "Red-White"
              }
              frame "Green-White" {
                # "Green-White"
              }
              frame "Blue-White" {
                # "Blue-White"
              }
              frame "Glow" {
              }
            }
            n151 = property class="IntGraph (strict)"(reference=w249, "ZScale.Maximum"=w250, "ZScale.MarkerVals[]"=w251) -> ()  [unwired: 1 in, 2 out]
          }
          frame "Graph Mode" {
            n152 = case shown="\"GetIntensity\"" "Graph Mode" {
              tunnel: w277 -> [w279 w283 w286 w289 w293]
              tunnel: w276 -> [_ _ _ _ w292]
              frame "FullChip" {
                n153 = for {
                  tunnel: w279 -> [w282] mode=indexing
                  n154 = property class="IntGraph (strict)"(reference=w282, "ActPaletteTool"=5 ("Palette:Active Tool"), "ZScale.ScaleFit"=u8 1 ("Z Scale.Scale Fit")) -> ()  [unwired: 1 in, 2 out]
                }
              }
              frame "ZoomIn" {
                n155 = for {
                  tunnel: w283 -> [w284] mode=indexing
                  n156 = property on="Property Node" class="IntGraph (strict)"(reference=w284, "ActPaletteTool"=6 ("Palette:Active Tool")) -> ()  [unwired: 1 in, 2 out]
                }
              }
              frame "ZoomOut" {
                n157 = for {
                  tunnel: w286 -> [w287] mode=indexing
                  n158 = property on="Property Node" class="IntGraph (strict)"(reference=w287, "ActPaletteTool"=7 ("Palette:Active Tool")) -> ()  [unwired: 1 in, 2 out]
                }
              }
              frame "Pan" {
                n159 = for {
                  tunnel: w289 -> [w290] mode=indexing
                  n160 = property on="Property Node" class="IntGraph (strict)"(reference=w290, "ActPaletteTool"=1 ("Palette:Active Tool")) -> ()  [unwired: 1 in, 2 out]
                }
              }
              frame "GetIntensity" {
                n161 = for {
                  tunnel: w293 -> [w300] mode=indexing
                  tunnel: w292 -> [w294]
                  i -> [w295]
                  n162 = property on="Property Node" class="IntGraph (strict)"(reference=w300, "ActPaletteTool"=0 ("Palette:Active Tool")) -> (reference out=w296:refnum<vi>)  [unwired: 1 in, 1 out]
                  n163 = To Long Integer(number=w294) -> (32bit integer=w299:i32)
                  n164 = Equal?(x=w299, y=w295) -> (x = y?=w298:bool)
                  n165 = property class="IntGraph (strict)"(reference=w296, "ZScale.Visible"=w298, "ZScale.Position"=T20 {"Left"=2275, "Top"=-325} ("Z Scale.Position")) -> ()  [unwired: 1 in, 2 out]
                }
              }
            }
          }
          frame "Active Channel" {
            n166 = for {
              tunnel: w303 -> [w308] mode=indexing
              tunnel: w302 -> [w307]
              i -> [w306]
              n167 = To Long Integer(number=w307) -> (32bit integer=w304:i32)
              n168 = Equal?(x=w304, y=w306) -> (x = y?=w305:bool)
              n169 = property class="IntGraph (strict)"(reference=w308, "ZScale.Visible"=w305, "ZScale.Position"=T20 {"Left"=2275, "Top"=-325} ("Z Scale.Position")) -> ()  [unwired: 1 in, 2 out]
            }
          }
          frame "Cursor" {
            w311 = 100.0 ("Cursor.Cursor Position:Cursor X")
            n170 = Index Array(array=w314, index=0) -> (element=w312:refnum<vi>)
            n171 = property class="IntGraph (strict)"(reference=w312, "Cursor.Visible"="Cursor", "Cursor.Cursor X"=w311, "Cursor.Cursor Y"=w311) -> ()  [unwired: 1 in, 2 out]
          }
        }
      }
      event Value Change {
        n172 = event-data() -> ("OldVal"=w327:T10, "NewVal"=w326:T10)  [unwired: 1 in, 4 out]
        n173 = property on="Graph Tools" class="Clust"() -> ("Controls[]"=w320:refnum<vi>[])  [unwired: 2 in, 2 out]
        n174 = Not Equal?(x=w327, y=w326) -> (x != y?=w325:T10)
        n175 = local read "Active Channel"() -> (w317:u16)
        n176 = Cluster To Array(cluster=w325) -> (array=w324:bool[])
        n177 = for {
          tunnel: w324 -> [w415] mode=indexing
          tunnel: w320 -> [w414] mode=indexing
          tunnel: [w414] -> w323
          stop <- w415 stop-if-true
        }
        n178 = To Long Integer(number=w317) -> (32bit integer=w321:i32)
        n179 = property class="Ctl"(reference=w323) -> (reference out=w316:refnum<vi>, "Label.Text"=w322:string)  [unwired: 1 in, 1 out]
        n180 = call "Graph Ref AE.vi"("Action"=enum16{"READ", "WRITE"}."READ") -> ("Graph Ref Out"=w318:refnum<vi>[])  [unwired: 10 in]
        n181 = case shown="\"Add Display\"" w322 {
          tunnel: w318 -> [_ w328 w341 w365 w370 _]
          tunnel: w321 -> [_ _ _ w364 w369 _]
          tunnel: w316 -> [_ _ _ _ _ w380]
          frame "False", Default {
          }
          frame "Add Display" {
            w331 = u16 0 items=["Read", "Write"] ("Action")
            w335 = u16 1 items=["Read", "Write"] ("Action")
            n182 = call "Arange_Displays_V2.vi"("Action"=w331) -> ("Number of Channels OUT"=w332:i32)  [unwired: 14 in]
            n183 = Increment(x=w332) -> (x+1=w334:i32)
            n184 = call "Arange_Displays_V2.vi"("Display References"=w328, "Action"=w335, "Number of Channels"=w334, "Aspect Ratio (h/w)"=1.0) -> ("Number of Channels OUT"=w329:i32)  [unwired: 11 in]
            n185 = for {
              N: w329 -> [_]
              tunnel: w328 -> [w340] mode=indexing
              tunnel: [w336] -> w330 mode=indexing
              i -> [w339]
              n186 = property class="IntGraph (strict)"(reference=w340) -> ("Label.Text"=w338:string)  [unwired: 1 in, 2 out]
              n187 = To Unsigned Word Integer(number=w339) -> (unsigned 16bit integer=w337:u16)
              n188 = Bundle("Label.Text"=w338, w337) -> (w336:cluster{"Label.Text":string, u16})  [unwired: 1 in]
            }
            n189 = property on="Active Channel" class="Ring (strict)"("StringsAndValues[]"=w330) -> ()  [unwired: 2 in, 2 out]
          }
          frame "Remove Display" {
            w344 = u16 0 items=["Read", "Write"] ("Action")
            w348 = u16 1 items=["Read", "Write"] ("Action")
            n190 = call "Arange_Displays_V2.vi"("Action"=w344) -> ("Number of Channels OUT"=w345:i32)  [unwired: 14 in]
            n191 = Decrement(x=w345) -> (x-1=w347:i32)
            n192 = call "Arange_Displays_V2.vi"("Display References"=w341, "Action"=w348, "Number of Channels"=w347, "Aspect Ratio (h/w)"=1.0) -> ("Number of Channels OUT"=w342:i32)  [unwired: 11 in]
            n193 = for {
              N: w342 -> [_]
              tunnel: w341 -> [w353] mode=indexing
              tunnel: [w349] -> w343 mode=indexing
              i -> [w352]
              n194 = property class="IntGraph (strict)"(reference=w353) -> ("Label.Text"=w351:string)  [unwired: 1 in, 2 out]
              n195 = To Unsigned Word Integer(number=w352) -> (unsigned 16bit integer=w350:u16)
              n196 = Bundle("Label.Text"=w351, w350) -> (w349:cluster{"Label.Text":string, u16})  [unwired: 1 in]
            }
            n197 = property on="Active Channel" class="Ring (strict)"("StringsAndValues[]"=w343) -> ()  [unwired: 2 in, 2 out]
          }
          frame "Load File" {
            w355 = u16 1 items=["Get Image", "Load and Read File"] ("Action")
            n198 = Index Array(array=w365, index=w364) -> (element=w354:refnum<vi>)
            n199 = call "OpenDBL.vi"("Action"=w355) -> ("Image"=w356:sgl[], "Dimensions (Z, Y, X, t)"=w357:i32[])  [unwired: 12 in, 1 out]
            n200 = Index Array(array=w357, index #1=1 ("index"), index #2=2 ("index")) -> (element #1=w360:i32, element #2=w361:i32)
            n201 = Reverse 1D Array(array=w356) -> (reversed array=w362:sgl[])
            n202 = Reshape Array(w362, w360, w361) -> (w363:sgl[][])
            n203 = property class="IntGraph (strict)"(reference=w354, "Value"=w363) -> ()  [unwired: 1 in, 2 out]
          }
          frame "Fit" {
            n204 = Index Array(array=w370, index=w369) -> (element=w368:refnum<vi>)
            n205 = local read "Image Acquisition Parameters"() -> (w367:T15)
            n206 = property class="IntGraph (strict)"(reference=w368) -> ("Value"=w376:sgl[][])  [unwired: 1 in, 2 out]
            n207 = vi-ref "QuickProfile_V3.vi"() -> (w371:refnum<vi>)
            n208 = property class="VI Interface Type 0"(reference=w371) -> ("Path"=w374:path)  [unwired: 1 in, 2 out]
            n209 = Unbundle By Name(w367) -> ("Pixel Size (nm)"=w366:dbl[])
            n210 = Index Array(array=w366, index=0) -> (element=w378:dbl)
            n211 = Open VI Reference(type specifier VI Refnum (for type only)=w371, vi path=w374, options=128) -> (vi reference=w372:refnum<vi>)  [unwired: 3 in, 1 out]
            n212 = call-by-ref "Start Asynchronous Call"(reference=w372, "Image IN"=w376, "Pixel Size (nm)"=w378) -> (reference out=w375:refnum<vi>)  [unwired: 15 in, 1 out]
            n213 = Close Reference(reference=w375) -> ()  [unwired: 1 in, 1 out]
          }
          frame "Single Screen" {
            n214 = property class="Ctl"(reference=w380) -> ("Value"=w379:variant)  [unwired: 1 in, 2 out]
            n215 = property class="App"() -> ("Disp.AllMonitors"=w384:T29)  [unwired: 2 in, 2 out]
            n216 = Variant To Data(type=FALSE, Variant=w379) -> (data=w381:bool)  [unwired: 1 in, 1 out]
            n217 = control-ref of="This VI"() -> (w383:refnum<vi>)
            n218 = case shown="True" w381 {
              tunnel: w384 -> [w388 w403]
              tunnel: T21 {"Left"=0, "Top"=0, "Right"=0, "Bottom"=0} ("FP Window Bounds 2") -> [w387 w402]
              tunnel: w383 -> [w386 w401]
              frame False {
                w397 = i16 0
                n219 = Index Array(array=w388, index #1=1 ("index"), index #2=0 ("index")) -> (element #1=w391:T30, element #2=w392:T30)
                n220 = Unbundle By Name(w392) -> ("Bounds.Left"=w394:i16, "Bounds.Bottom"=w395:i16, "Bounds.Top"=w396:i16)
                n221 = Unbundle By Name(w391) -> ("Bounds.Right"=w393:i16)
                n222 = Subtract(x=w393, y=w394) -> (x-y=w398:i16)
                n223 = Subtract(x=w395, y=w396) -> (x-y=w399:i16)
                n224 = Bundle By Name(cluster=w387, "Left"=w397, "Top"=w397, "Right"=w398, "Bottom"=w399) -> (w400:T21)
                n225 = property class="VI"(reference=w386, "Front Panel.WinBounds"=w400) -> ()  [unwired: 1 in, 2 out]
              }
              frame True {
                w406 = i16 0
                n226 = Index Array(array=w403, index=0) -> (element=w410:T30)
                n227 = Unbundle By Name(w410) -> ("Bounds.Right"=w411:i16, "Bounds.Bottom"=w408:i16, "Bounds.Top"=w407:i16)
                n228 = Subtract(x=w408, y=w407) -> (x-y=w405:i16)
                n229 = Bundle By Name(cluster=w402, "Left"=w406, "Top"=w406, "Right"=w411, "Bottom"=w405) -> (w404:T21)
                n230 = property class="VI"(reference=w401, "Front Panel.WinBounds"=w404) -> (reference out=w413:refnum<vi>)  [unwired: 1 in, 1 out]
                n231 = property class="VI"(reference=w413, "FP.State"=T22."Maximized" ("Front Panel Window:State")) -> ()  [unwired: 1 in, 2 out]
              }
            }
          }
        }
      }
      event "SLM", "Timing", "DM": Value Change {
        n232 = event-data() -> ("CtlRef"=w419:refnum<vi>, "NewVal"=w416:bool)  [unwired: 1 in, 1 out]
        n233 = property class="Bool (strict)"(reference=w419) -> ("Label.Text"=w418:string)  [unwired: 1 in, 2 out]
        n234 = case shown="\"SLM\", Default" w418 {
          tunnel: w416 -> [w420 w434 w448]
          frame "SLM", Default {
            n235 = case shown="False" w420 {
              frame False {
                n236 = To Variant(anything=TRUE) -> (Variant=w426:variant)
                n237 = call "SLM AE.vi"("Action"=enum16{"READ", "WRITE"}."READ") -> ("SLM Ref Out"=w427:refnum<vi>)  [unwired: 10 in]
                n238 = invoke class="VI" method="Ctrl Val.Set"(reference=w427, "Control Name"="Exit", "Value"=w426) -> (reference out=w423:refnum<vi>, error out=w422:errorcluster)  [unwired: 2 in, 3 out]
                n239 = invoke on="Hamamatsu LCOS" class="SubPnl" method="Remove VI"(error in=w422) -> (error out=w421:errorcluster)  [unwired: 2 in, 2 out]
                n240 = Close Reference(reference=w423, error in (no error)=w421) -> ()  [unwired: 1 out]
              }
              frame True {
                n241 = Open VI Reference(vi path=path "C:/Users/ED STED/Documents/Test Control Software/Host VIs/SLM/SLM Control.vi") -> (vi reference=w432:refnum<vi>)  [unwired: 5 in, 1 out]
                n242 = invoke class="VI" method="Run VI"(reference=w432, "Wait until done"=FALSE ("Wait Until Done")) -> (reference out=w429:refnum<vi>)  [unwired: 3 in, 4 out]
                n243 = invoke on="Hamamatsu LCOS" class="SubPanel" method="Insert VI"("VI Ref"=w429) -> ()  [unwired: 3 in, 4 out]
                n244 = call "SLM AE.vi"("Action"=enum16{"READ", "WRITE"}."WRITE", "SLM Ref In"=w429) -> ()  [unwired: 9 in, 1 out]
              }
            }
          }
          frame "DM" {
            n245 = case shown="True" w434 {
              frame False {
                n246 = call "DM_Ref_AE.vi"("Action"=enum16{"READ", "WRITE"}."READ") -> ("DM Ref Out"=w441:refnum<vi>)  [unwired: 10 in]
                n247 = To Variant(anything=TRUE) -> (Variant=w440:variant)
                n248 = invoke class="VI" method="Ctrl Val.Set"(reference=w441, "Control Name"="Exit", "Value"=w440) -> (reference out=w437:refnum<vi>, error out=w436:errorcluster)  [unwired: 2 in, 3 out]
                n249 = invoke on="Hamamatsu LCOS" class="SubPnl" method="Remove VI"(error in=w436) -> (error out=w435:errorcluster)  [unwired: 2 in, 2 out]
                n250 = Close Reference(reference=w437, error in (no error)=w435) -> ()  [unwired: 1 out]
              }
              frame True {
                n251 = Open VI Reference(vi path=path "C:/Users/ED STED/Documents/Test Control Software/Host VIs/DM/DM_Control_STED.vi") -> (vi reference=w446:refnum<vi>)  [unwired: 5 in, 1 out]
                n252 = invoke class="VI" method="Run VI"(reference=w446, "Wait until done"=FALSE ("Wait Until Done")) -> (reference out=w443:refnum<vi>)  [unwired: 3 in, 4 out]
                n253 = invoke on="BM Multi" class="SubPanel" method="Insert VI"("VI Ref"=w443) -> ()  [unwired: 3 in, 4 out]
                n254 = call "DM_Ref_AE.vi"("Action"=enum16{"READ", "WRITE"}."WRITE", "DM Ref In"=w443) -> ()  [unwired: 9 in, 1 out]
              }
            }
          }
          frame "Timing" {
            n255 = case shown="True" w448 {
              frame False {
                n256 = To Variant(anything=TRUE) -> (Variant=w453:variant)
                n257 = call "GateDelay AE.vi"("Action"=enum16{"READ", "WRITE"}."READ") -> ("Gate Delay Ref Out"=w454:refnum<vi>)  [unwired: 10 in]
                n258 = invoke class="VI" method="Ctrl Val.Set"(reference=w454, "Control Name"="Exit", "Value"=w453) -> (reference out=w449:refnum<vi>, error out=w450:errorcluster)  [unwired: 2 in, 3 out]
                n259 = invoke on="Timing" class="SubPnl" method="Remove VI"(error in=w450) -> (error out=w456:errorcluster)  [unwired: 2 in, 2 out]
                n260 = Close Reference(reference=w449, error in (no error)=w456) -> ()  [unwired: 1 out]
              }
              frame True {
                n261 = Open VI Reference(vi path=path "C:/Users/ED STED/Documents/Test Control Software/Host VIs/Time Delay/GateDelay_Control_V1.vi") -> (vi reference=w459:refnum<vi>)  [unwired: 5 in, 1 out]
                n262 = invoke class="VI" method="Run VI"(reference=w459, "Wait until done"=FALSE ("Wait Until Done")) -> (reference out=w458:refnum<vi>)  [unwired: 3 in, 4 out]
                n263 = invoke on="Timing" class="SubPanel" method="Insert VI"("VI Ref"=w458) -> ()  [unwired: 3 in, 4 out]
                n264 = call "GateDelay AE.vi"("Action"=enum16{"READ", "WRITE"}."WRITE", "Gate Delay Ref In"=w458) -> ()  [unwired: 9 in, 1 out]
              }
            }
          }
        }
      }
      event Value Change {
        n265 = event-data() -> ("CtlRef"=w467:refnum<vi>)  [unwired: 1 in, 2 out]
        n266 = property class="Ctl"(reference=w467) -> ("Label.Text"=w466:string)  [unwired: 1 in, 2 out]
        n267 = call "Image Aquisition Param Ctrl_AE.vi"("Action"=enum16{"READ", "WRITE"}."READ") -> ("Image Acquisition Parameters Out"=w464:T15)  [unwired: 10 in]
        n268 = control-ref of="Abort AllStage"() -> (w462:refnum<vi>)
        n269 = case shown="\"ZoomDown\"" w466 {
          tunnel: w464 -> [w470 w476 w545 _]
          tunnel: "Focus Control" -> [_ w471 w540 w612]
          tunnel: w462 -> [_ w472 w541 w611]
          frame "SetZoom", Default {
            n270 = control-ref of="Channel 1"() -> (w469:refnum<vi>)
            n271 = call "Set_Focus_Plane.vi"("Image Acquisition Parameters Out"=w470, "IntensityGraph in"=w469) -> ()  [unwired: 10 in]
          }
          frame "ZoomUp" {
            n272 = Unbundle By Name(w471) -> ("ZoomStepI16"=w473:enum16{"Coarse", "Medium", "Fine"})
            n273 = Unbundle By Name(w476) -> ("Scan Type"=w475:enum16{"Sample Scanning", "Beam Scanning"}, "Scan Mode"=w474:enum16{"XY", "XZ", "YZ", "XYZ"})
            n274 = flat-sequence {
              tunnel: w475 -> [w484]
              tunnel: w474 -> [w483]
              tunnel: w473 -> [w482]
              tunnel: w472 -> [w539]
              tunnel: w471 -> [w533]
              frame #0 {
                n275 = case shown="\"Medium\"" w482 {
                  tunnel: [i16 500 i16 150 i16 50] -> w480
                  frame "Coarse", Default {
                  }
                  frame "Medium" {
                  }
                  frame "Fine" {
                  }
                }
                n276 = call "Manual Controls Action Engine.vi"("Action"=enum16{"Read", "Write"}."Read") -> ("Manual Controls Out"=w481:T18)  [unwired: 14 in]
                n277 = case shown="\"Beam Scanning\"" w484 {
                  tunnel: w483 -> [w498 w524]
                  tunnel: w481 -> [w497 w523]
                  tunnel: w480 -> [w496 w522]
                  tunnel: [w495 w519] -> w479
                  frame "Sample Scanning", Default {
                    n278 = case shown="\"YZ\"" w498 {
                      tunnel: w497 -> [w503 w508 w513 w518]
                      tunnel: w496 -> [w501 w506 w511 w516]
                      tunnel: [w500 w505 w510 w515] -> w495
                      tunnel: [w499 w504 w509 w514] -> w492
                      frame "XZ" {
                        n279 = Unbundle By Name(w503) -> ("Y Axis Voltage (I16)"=w502:i16)
                        n280 = Add(x=w502, y=w501) -> (x+y=w499:i16)
                        n281 = Bundle By Name(cluster=w503, "Y Axis Voltage (I16)"=w499) -> (w500:T18)
                      }
                      frame "YZ" {
                        n282 = Unbundle By Name(w508) -> ("X Axis Voltage (I16)"=w507:i16)
                        n283 = Add(x=w507, y=w506) -> (x+y=w504:i16)
                        n284 = Bundle By Name(cluster=w508, "X Axis Voltage (I16)"=w504) -> (w505:T18)
                      }
                      frame "XYZ" {
                        n285 = Unbundle By Name(w513) -> ("Z Axis Voltage (I16)"=w512:i16)
                        n286 = Add(x=w512, y=w511) -> (x+y=w509:i16)
                        n287 = Bundle By Name(cluster=w513, "Z Axis Voltage (I16)"=w509) -> (w510:T18)
                      }
                      frame "XY" {
                        n288 = Unbundle By Name(w518) -> ("Z Axis Voltage (I16)"=w517:i16)
                        n289 = Add(x=w517, y=w516) -> (x+y=w514:i16)
                        n290 = Bundle By Name(cluster=w518, "Z Axis Voltage (I16)"=w514) -> (w515:T18)
                      }
                    }
                    n291 = call "FPGA-7842R-Control V1.vi"("Action"=FPGA-7842R-Reference."Unused Axis I16", "Initialize"=TRUE, "Unused Axis Offset (I16)"=w492) -> ()  [unwired: 11 in, 2 out]
                    n292 = call "Scan Parameters Action Engine.vi"("Action"=enum16{"Read", "Write"}."Read") -> ("Scan Parameters OUT"=w491:T17)  [unwired: 14 in]
                    n293 = Bundle By Name(cluster=w491, "Unused_Axis_I16"=w492) -> (w490:T17)
                    n294 = call "Scan Parameters Action Engine.vi"("Action"=enum16{"Read", "Write"}."Write", "Scan Parameters IN"=w490) -> ()  [unwired: 13 in, 1 out]
                  }
                  frame "Beam Scanning" {
                    n295 = case shown="\"XY\", Default" w524 {
                      tunnel: w523 -> [w529]
                      tunnel: w522 -> [w527]
                      tunnel: [w526] -> w519
                      frame "XY", Default {
                        n296 = Unbundle By Name(w529) -> ("Z Axis Voltage (I16)"=w528:i16)
                        n297 = Add(x=w528, y=w527) -> (x+y=w525:i16)
                        n298 = Bundle By Name(cluster=w529, "Z Axis Voltage (I16)"=w525) -> (w526:T18)
                      }
                    }
                    n299 = call "FPGA-7842R-Control V1.vi"("Action"=FPGA-7842R-Reference."Stage Control", "Manual Controls"=w519, "Initialize"=TRUE) -> ()  [unwired: 11 in, 2 out]
                  }
                }
                n300 = call "Manual Controls Action Engine.vi"("Action"=enum16{"Read", "Write"}."Write", "Manual Controls In"=w479) -> ()  [unwired: 13 in, 1 out]
              }
              frame #1 {
                n301 = call "AE_AllStages_Action V2.vi"("Abort"=w539, "Axis"=bool[] [TRUE, TRUE, TRUE], "Stage ID"="P612", "Action"=StageStates."POSITION") -> ("Position Out"=w535:dbl[])  [unwired: 5 in, 2 out]
                n302 = Index Array(array=w535, index=2) -> (element=w532:dbl)
                n303 = Bundle By Name(cluster=w533, "Z Position"=w532, "ZoomUp"=FALSE) -> (w531:T12)
                n304 = property on="Focus Control" class="Clust"("Value"=w531) -> ()  [unwired: 2 in, 2 out]
              }
            }
          }
          frame "ZoomDown" {
            n305 = Unbundle By Name(w545) -> ("Scan Type"=w544:enum16{"Sample Scanning", "Beam Scanning"}, "Scan Mode"=w543:enum16{"XY", "XZ", "YZ", "XYZ"})
            n306 = Unbundle By Name(w540) -> ("ZoomStepI16"=w542:enum16{"Coarse", "Medium", "Fine"})
            n307 = flat-sequence {
              tunnel: w544 -> [w554]
              tunnel: w543 -> [w553]
              tunnel: w542 -> [w552]
              tunnel: w541 -> [w607]
              tunnel: w540 -> [w604]
              frame #0 {
                n308 = case shown="\"Fine\"" w552 {
                  tunnel: [i16 500 i16 150 i16 50] -> w548
                  frame "Coarse", Default {
                  }
                  frame "Medium" {
                  }
                  frame "Fine" {
                  }
                }
                n309 = call "Manual Controls Action Engine.vi"("Action"=enum16{"Read", "Write"}."Read") -> ("Manual Controls Out"=w550:T18)  [unwired: 14 in]
                n310 = Negate(x=w548) -> (-x=w546:i16)
                n311 = case shown="Default" w554 {
                  tunnel: w553 -> [w568 w594 _]
                  tunnel: w550 -> [w567 w593 w600]
                  tunnel: w546 -> [w566 w592 _]
                  tunnel: [w565 w589 w600] -> w547
                  frame "Sample Scanning" {
                    n312 = case shown="\"XYZ\"" w568 {
                      tunnel: w567 -> [w573 w578 w583 w588]
                      tunnel: w566 -> [w571 w576 w581 w586]
                      tunnel: [w570 w575 w580 w585] -> w565
                      tunnel: [w569 w574 w579 w584] -> w558
                      frame "XZ" {
                        n313 = Unbundle By Name(w573) -> ("Y Axis Voltage (I16)"=w572:i16)
                        n314 = Add(x=w572, y=w571) -> (x+y=w569:i16)
                        n315 = Bundle By Name(cluster=w573, "Y Axis Voltage (I16)"=w569) -> (w570:T18)
                      }
                      frame "YZ" {
                        n316 = Unbundle By Name(w578) -> ("X Axis Voltage (I16)"=w577:i16)
                        n317 = Add(x=w577, y=w576) -> (x+y=w574:i16)
                        n318 = Bundle By Name(cluster=w578, "X Axis Voltage (I16)"=w574) -> (w575:T18)
                      }
                      frame "XYZ" {
                        n319 = Unbundle By Name(w583) -> ("Z Axis Voltage (I16)"=w582:i16)
                        n320 = Add(x=w582, y=w581) -> (x+y=w579:i16)
                        n321 = Bundle By Name(cluster=w583, "Z Axis Voltage (I16)"=w579) -> (w580:T18)
                      }
                      frame "XY" {
                        n322 = Unbundle By Name(w588) -> ("Z Axis Voltage (I16)"=w587:i16)
                        n323 = Add(x=w587, y=w586) -> (x+y=w584:i16)
                        n324 = Bundle By Name(cluster=w588, "Z Axis Voltage (I16)"=w584) -> (w585:T18)
                      }
                    }
                    n325 = call "FPGA-7842R-Control V1.vi"("Action"=FPGA-7842R-Reference."Unused Axis I16", "Initialize"=TRUE, "Unused Axis Offset (I16)"=w558) -> ()  [unwired: 11 in, 2 out]
                    n326 = call "Scan Parameters Action Engine.vi"("Action"=enum16{"Read", "Write"}."Read") -> ("Scan Parameters OUT"=w561:T17)  [unwired: 14 in]
                    n327 = Bundle By Name(cluster=w561, "Unused_Axis_I16"=w558) -> (w562:T17)
                    n328 = call "Scan Parameters Action Engine.vi"("Action"=enum16{"Read", "Write"}."Write", "Scan Parameters IN"=w562) -> ()  [unwired: 13 in, 1 out]
                  }
                  frame "Beam Scanning" {
                    n329 = case shown="\"XY\", Default" w594 {
                      tunnel: w593 -> [w599]
                      tunnel: w592 -> [w597]
                      tunnel: [w596] -> w589
                      tunnel: [w595] -> _
                      frame "XY", Default {
                        n330 = Unbundle By Name(w599) -> ("Z Axis Voltage (I16)"=w598:i16)
                        n331 = Add(x=w598, y=w597) -> (x+y=w595:i16)
                        n332 = Bundle By Name(cluster=w599, "Z Axis Voltage (I16)"=w595) -> (w596:T18)
                      }
                    }
                    n333 = call "FPGA-7842R-Control V1.vi"("Action"=FPGA-7842R-Reference."Stage Control", "Manual Controls"=w589, "Initialize"=TRUE) -> ()  [unwired: 11 in, 2 out]
                  }
                  frame Default {
                  }
                }
                n334 = call "Manual Controls Action Engine.vi"("Action"=enum16{"Read", "Write"}."Write", "Manual Controls In"=w547) -> ()  [unwired: 13 in, 1 out]
              }
              frame #1 {
                n335 = call "AE_AllStages_Action V2.vi"("Abort"=w607, "Axis"=bool[] [TRUE, TRUE, TRUE], "Stage ID"="P612", "Action"=StageStates."POSITION") -> ("Position Out"=w606:dbl[])  [unwired: 5 in, 2 out]
                n336 = Index Array(array=w606, index=2) -> (element=w603:dbl)
                n337 = Bundle By Name(cluster=w604, "Z Position"=w603, "ZoomDown"=FALSE) -> (w602:T12)
                n338 = property on="Focus Control" class="Clust"("Value"=w602) -> ()  [unwired: 2 in, 2 out]
              }
            }
          }
          frame "Z Position" {
            n339 = flat-sequence {
              tunnel: w612 -> [w623]
              tunnel: w611 -> [w625]
              frame #0 {
                n340 = Unbundle By Name(w623) -> ("Z Position"=w621:dbl)
                n341 = call "Manual Controls Action Engine.vi"("Action"=enum16{"Read", "Write"}."Read") -> ("Manual Controls Out"=w617:T18)  [unwired: 14 in]
                n342 = Divide(x=w621, y=10.0) -> (x/y=w619:dbl)
                n343 = call "Volts to I16.vi"("Voltage (V)"=w619) -> ("I16"=w618:i16)  [unwired: 13 in, 1 out]
                n344 = Bundle By Name(cluster=w617, "Z Axis Voltage (I16)"=w618) -> (w613:T18)
                n345 = call "Manual Controls Action Engine.vi"("Action"=enum16{"Read", "Write"}."Write", "Manual Controls In"=w613) -> ()  [unwired: 13 in, 1 out]
                n346 = call "FPGA-7842R-Control V1.vi"("Action"=FPGA-7842R-Reference."Stage Control", "Manual Controls"=w613, "Initialize"=TRUE) -> ()  [unwired: 11 in, 2 out]
              }
              frame #1 {
                n347 = call "AE_AllStages_Action V2.vi"("Abort"=w625, "Axis"=bool[] [TRUE, TRUE, TRUE], "Stage ID"="P612", "Action"=StageStates."POSITION") -> ("Position Out"=w627:dbl[])  [unwired: 5 in, 2 out]
                n348 = Index Array(array=w627, index=2) -> (element=w624:dbl)
              }
            }
          }
        }
      }
      event Value Change {
        n349 = event-data() -> ("CtlRef"=w642:refnum<vi>)  [unwired: 1 in, 2 out]
        n350 = property class="Bool"(reference=w642) -> ("Label.Text"=w641:string)  [unwired: 1 in, 2 out]
        n351 = Unbundle By Name("Micrometer Sample Stage Holder Z - M227") -> ("Step Size (mm)"=w640:dbl)
        n352 = Build Array(w640, w640, w640) -> (w637:dbl[])
        n353 = case shown="\"Up_M227\"" w641 {
          tunnel: w637 -> [w645 w646]
          tunnel: [w643 w646] -> w636
          frame "Down_M227", Default {
            n354 = Subtract(x=dbl[] [0.0, 0.0, 0.0], y=w645) -> (x-y=w643:dbl[])
          }
          frame "Up_M227" {
          }
        }
        n355 = control-ref of="Abort AllStage"() -> (w639:refnum<vi>)
        n356 = call "AE_AllStages_Action V2.vi"("Velocity"=0.3, "Abort"=w639, "Positions"=w636, "Axis"=bool[] [TRUE, TRUE, TRUE], "Stage ID"="M227", "Action"=StageStates."MVR") -> ()  [unwired: 3 in, 3 out]
      }
      event Value Change {
        n357 = event-data() -> ("CtlRef"=w656:refnum<vi>)  [unwired: 1 in, 2 out]
        n358 = Unbundle By Name("Upper Objective Holder Z - N664 (8~19 mm)") -> ("Position"=w650:dbl, "Step Size (um)"=w651:dbl)
        n359 = property class="Ctl"(reference=w656) -> ("Label.Text"=w655:string)  [unwired: 1 in, 2 out]
        n360 = Divide(x=w651, y=1000.0) -> (x/y=w653:dbl)
        n361 = Build Array(w650) -> (w649:dbl[])
        n362 = Build Array(w653) -> (w652:dbl[])
        n363 = case shown="\"Up_N664\"" w655 {
          tunnel: w652 -> [w660 _ w686]
          tunnel: "Upper Objective Holder Z - N664 (8~19 mm)" -> [w657 _ w683]
          tunnel: w649 -> [_ w677 _]
          frame "Down_N664" {
            n364 = flat-sequence {
              tunnel: w660 -> [w661]
              tunnel: [w663] -> w659
              tunnel: [w662] -> w658
              tunnel: w659 -> [w670]
              tunnel: w658 -> [w669]
              tunnel: w657 -> [w668]
              frame #0 {
                w663 = bool[] [TRUE] ("Axis")
                n365 = control-ref of="Abort AllStage"() -> (w662:refnum<vi>)
                n366 = call "AE_AllStages_Action V2.vi"("Velocity"=1.0, "Abort"=w662, "Positions"=w661, "Axis"=w663, "Stage ID"="N664", "Action"=StageStates."MVR") -> ()  [unwired: 3 in, 3 out]
              }
              frame #1 {
                n367 = call "AE_AllStages_Action V2.vi"("Abort"=w669, "Axis"=w670, "Stage ID"="N664", "Action"=StageStates."POSITION") -> ("Position Out"=w674:dbl[])  [unwired: 5 in, 2 out]
                n368 = Index Array(array=w674, index=0) -> (element=w672:dbl)
                n369 = Bundle By Name(cluster=w668, "Position"=w672, "Down_N664"=FALSE ("Up_N664")) -> (w667:T5)
                n370 = property on="Upper Objective Holder Z - N664 (8~19 mm)" class="Clust"("Value"=w667) -> ()  [unwired: 2 in, 2 out]
              }
            }
          }
          frame "Position", Default {
            n371 = control-ref of="Abort AllStage"() -> (w681:refnum<vi>)
            n372 = call "AE_AllStages_Action V2.vi"("Velocity"=1.0, "Abort"=w681, "Positions"=w677, "Axis"=bool[] [TRUE, TRUE, TRUE], "Stage ID"="N664", "Action"=StageStates."MOVE") -> ()  [unwired: 3 in, 3 out]
          }
          frame "Up_N664" {
            n373 = flat-sequence {
              tunnel: w686 -> [w689]
              tunnel: [w691] -> w685
              tunnel: [w690] -> w684
              tunnel: w685 -> [w704]
              tunnel: w684 -> [w701]
              tunnel: w683 -> [w698]
              frame #0 {
                w690 = bool[] [TRUE] ("Axis")
                n374 = Subtract(x=dbl[] [0.0], y=w689) -> (x-y=w687:dbl[])
                n375 = control-ref of="Abort AllStage"() -> (w691:refnum<vi>)
                n376 = call "AE_AllStages_Action.vi"("Velocity"=1.0, "Abort"=w691, "Positions"=w687, "Axis"=w690, "Stage ID"="N664", "Action"=StageStates."MVR") -> ()  [unwired: 3 in, 3 out]
              }
              frame #1 {
                n377 = call "AE_AllStages_Action V2.vi"("Abort"=w704, "Axis"=w701, "Stage ID"="N664", "Action"=StageStates."POSITION") -> ("Position Out"=w700:dbl[])  [unwired: 5 in, 2 out]
                n378 = Index Array(array=w700, index=0) -> (element=w696:dbl)
                n379 = Bundle By Name(cluster=w698, "Position"=w696, "Up_N664"=FALSE) -> (w697:T5)
                n380 = property on="Upper Objective Holder Z - N664 (8~19 mm)" class="Clust"("Value"=w697) -> ()  [unwired: 2 in, 2 out]
              }
            }
          }
        }
      }
      event Value Change {
        n381 = event-data() -> ("CtlRef"=w711:refnum<vi>)  [unwired: 1 in, 2 out]
        n382 = property class="Ctl"(reference=w711) -> ("Label.Text"=w710:string)  [unwired: 1 in, 2 out]
        n383 = Unbundle By Name("Bottom Objective Holder XY - P612 (0~100 um)") -> ("Step Size (um)"=w709:dbl, "X"=w708:dbl, "Y"=w707:dbl)
        n384 = case shown="\"Up Button\"" w710 {
          tunnel: w709 -> [w712 w737 w760 w786 w811 w836 w863 w894]
          tunnel: w708 -> [_ _ _ _ _ w832 w859 _]
          tunnel: w707 -> [_ _ _ _ _ w831 w858 _]
          frame "Home Button", Default {
            n385 = flat-sequence {
              tunnel: [w718] -> w715
              tunnel: [w717] -> w714
              tunnel: [w716] -> w713
              tunnel: w712 -> [w716]
              tunnel: w715 -> [w732]
              tunnel: w714 -> [w731]
              tunnel: w713 -> [w724]
              frame #0 {
                w718 = bool[] [TRUE, TRUE] ("Axis")
                n386 = control-ref of="Abort AllStage"() -> (w717:refnum<vi>)
                n387 = call "AE_AllStages_Action V2.vi"("Velocity"=3.0, "Abort"=w717, "Positions"=dbl[] [50.0, 50.0], "Axis"=w718, "Stage ID"="P612", "Action"=StageStates."MOVE") -> ()  [unwired: 3 in, 3 out]
              }
              frame #1 {
                w727 = FALSE
                n388 = call "AE_AllStages_Action V2.vi"("Abort"=w731, "Axis"=w732, "Stage ID"="P612", "Action"=StageStates."POSITION") -> ("Position Out"=w729:dbl[])  [unwired: 5 in, 2 out]
                n389 = Index Array(array=w729, index=0) -> (element=w726:dbl)
                n390 = Index Array(array=w729, index=1) -> (element=w725:dbl)
                n391 = Bundle(w727, w727, w727, w727, w727, "Step Size (um)"=w724, "Numeric"=w726, "Numeric"=w725) -> (w723:T31)  [unwired: 1 in]
                n392 = property on="Bottom Objective Holder XY - P612 (0~100 um)" class="Clust"("Value"=w723) -> ()  [unwired: 2 in, 2 out]
              }
            }
          }
          frame "Up Button" {
            n393 = flat-sequence {
              tunnel: w737 -> [w739]
              tunnel: [w742] -> w736
              tunnel: [w739] -> w735
              tunnel: w736 -> [w749]
              tunnel: w735 -> [w748]
              frame #0 {
                n394 = control-ref of="Abort AllStage"() -> (w742:refnum<vi>)
                n395 = Build Array(0.0 ("element"), w739) -> (w740:dbl[])
                n396 = call "AE_AllStages_Action V2.vi"("Velocity"=3.0, "Abort"=w742, "Positions"=w740, "Axis"=bool[] [TRUE, TRUE], "Stage ID"="P612", "Action"=StageStates."MVR") -> ()  [unwired: 3 in, 3 out]
              }
              frame #1 {
                w752 = FALSE
                n397 = call "AE_AllStages_Action V2.vi"("Abort"=w749, "Axis"=bool[] [TRUE, TRUE], "Stage ID"="P612", "Action"=StageStates."POSITION") -> ("Position Out"=w754:dbl[])  [unwired: 5 in, 2 out]
                n398 = Index Array(array=w754, index=0) -> (element=w751:dbl)
                n399 = Index Array(array=w754, index=1) -> (element=w750:dbl)
                n400 = Bundle(w752, w752, w752, w752, w752, "Step Size (um)"=w748, "Numeric"=w751, "Numeric"=w750) -> (w747:T31)  [unwired: 1 in]
                n401 = property on="Bottom Objective Holder XY - P612 (0~100 um)" class="Clust"("Value"=w747) -> ()  [unwired: 2 in, 2 out]
              }
            }
          }
          frame "Down Button" {
            n402 = flat-sequence {
              tunnel: w760 -> [w764]
              tunnel: [w767] -> w759
              tunnel: [w764] -> w758
              tunnel: w759 -> [w774]
              tunnel: w758 -> [w773]
              frame #0 {
                n403 = control-ref of="Abort AllStage"() -> (w767:refnum<vi>)
                n404 = Subtract(x=0.0, y=w764) -> (x-y=w762:dbl)
                n405 = Build Array(0.0 ("element"), w762) -> (w765:dbl[])
                n406 = call "AE_AllStages_Action V2.vi"("Velocity"=3.0, "Abort"=w767, "Positions"=w765, "Axis"=bool[] [TRUE, TRUE], "Stage ID"="P612", "Action"=StageStates."MVR") -> ()  [unwired: 3 in, 3 out]
              }
              frame #1 {
                w777 = FALSE
                n407 = call "AE_AllStages_Action V2.vi"("Abort"=w774, "Axis"=bool[] [TRUE, TRUE], "Stage ID"="P612", "Action"=StageStates."POSITION") -> ("Position Out"=w779:dbl[])  [unwired: 5 in, 2 out]
                n408 = Index Array(array=w779, index=0) -> (element=w776:dbl)
                n409 = Index Array(array=w779, index=1) -> (element=w775:dbl)
                n410 = Bundle(w777, w777, w777, w777, w777, "Step Size (um)"=w773, "Numeric"=w776, "Numeric"=w775) -> (w772:T31)  [unwired: 1 in]
                n411 = property on="Bottom Objective Holder XY - P612 (0~100 um)" class="Clust"("Value"=w772) -> ()  [unwired: 2 in, 2 out]
              }
            }
          }
          frame "Left Button" {
            n412 = flat-sequence {
              tunnel: w786 -> [w789]
              tunnel: [w792] -> w785
              tunnel: [w791] -> w784
              tunnel: [w789] -> w783
              tunnel: w785 -> [w799]
              tunnel: w784 -> [w798]
              tunnel: w783 -> [w797]
              frame #0 {
                w791 = bool[] [TRUE, FALSE] ("Axis")
                n413 = control-ref of="Abort AllStage"() -> (w792:refnum<vi>)
                n414 = Subtract(x=0.0, y=w789) -> (x-y=w787:dbl)
                n415 = Build Array(w787) -> (w790:dbl[])
                n416 = call "AE_AllStages_Action V2.vi"("Velocity"=3.0, "Abort"=w792, "Positions"=w790, "Axis"=w791, "Stage ID"="P612", "Action"=StageStates."MVR") -> ()  [unwired: 3 in, 3 out]
              }
              frame #1 {
                w802 = FALSE
                n417 = call "AE_AllStages_Action V2.vi"("Abort"=w799, "Axis"=w798, "Stage ID"="P612", "Action"=StageStates."POSITION") -> ("Position Out"=w804:dbl[])  [unwired: 5 in, 2 out]
                n418 = Index Array(array=w804, index=0) -> (element=w801:dbl)
                n419 = Index Array(array=w804, index=1) -> (element=w800:dbl)
                n420 = Bundle(w802, w802, w802, w802, w802, "Step Size (um)"=w797, "Numeric"=w801, "Numeric"=w800) -> (w796:T31)  [unwired: 1 in]
                n421 = property on="Bottom Objective Holder XY - P612 (0~100 um)" class="Clust"("Value"=w796) -> ()  [unwired: 2 in, 2 out]
              }
            }
          }
          frame "Right Button" {
            n422 = flat-sequence {
              tunnel: w811 -> [w812]
              tunnel: [w815] -> w810
              tunnel: [w814] -> w809
              tunnel: [w812] -> w808
              tunnel: w810 -> [w822]
              tunnel: w809 -> [w821]
              tunnel: w808 -> [w820]
              frame #0 {
                w814 = bool[] [TRUE, FALSE] ("Axis")
                n423 = control-ref of="Abort AllStage"() -> (w815:refnum<vi>)
                n424 = Build Array(w812) -> (w813:dbl[])
                n425 = call "AE_AllStages_Action V2.vi"("Velocity"=3.0, "Abort"=w815, "Positions"=w813, "Axis"=w814, "Stage ID"="P612", "Action"=StageStates."MVR") -> ()  [unwired: 3 in, 3 out]
              }
              frame #1 {
                w825 = FALSE
                n426 = call "AE_AllStages_Action V2.vi"("Abort"=w822, "Axis"=w821, "Stage ID"="P612", "Action"=StageStates."POSITION") -> ("Position Out"=w827:dbl[])  [unwired: 5 in, 2 out]
                n427 = Index Array(array=w827, index=0) -> (element=w824:dbl)
                n428 = Index Array(array=w827, index=1) -> (element=w823:dbl)
                n429 = Bundle(w825, w825, w825, w825, w825, "Step Size (um)"=w820, "Numeric"=w824, "Numeric"=w823) -> (w819:T31)  [unwired: 1 in]
                n430 = property on="Bottom Objective Holder XY - P612 (0~100 um)" class="Clust"("Value"=w819) -> ()  [unwired: 2 in, 2 out]
              }
            }
          }
          frame "X" {
            n431 = flat-sequence {
              tunnel: w836 -> [w840]
              tunnel: [w842] -> w835
              tunnel: [w841] -> w834
              tunnel: [w840] -> w833
              tunnel: w832 -> [w839]
              tunnel: w831 -> [w838]
              tunnel: w835 -> [w852]
              tunnel: w834 -> [w851]
              tunnel: w833 -> [w850]
              frame #0 {
                w841 = bool[] [TRUE, TRUE] ("Axis")
                n432 = control-ref of="Abort AllStage"() -> (w842:refnum<vi>)
                n433 = Build Array(w839, w838) -> (w837:dbl[])
                n434 = call "AE_AllStages_Action V2.vi"("Velocity"=3.0, "Abort"=w842, "Positions"=w837, "Axis"=w841, "Stage ID"="P612", "Action"=StageStates."MOVE") -> ()  [unwired: 3 in, 3 out]
              }
              frame #1 {
                w854 = FALSE
                n435 = call "AE_AllStages_Action V2.vi"("Abort"=w852, "Axis"=w851, "Stage ID"="P612", "Action"=StageStates."POSITION") -> ("Position Out"=w846:dbl[])  [unwired: 5 in, 2 out]
                n436 = Index Array(array=w846, index #1=0 ("index"), index #2=1 ("index")) -> (element #1=w853:dbl, element #2=w847:dbl)
                n437 = Bundle(w854, w854, w854, w854, w854, "Step Size (um)"=w850, "Numeric"=w853, "Numeric"=w847) -> (w849:T31)  [unwired: 1 in]
                n438 = property on="Bottom Objective Holder XY - P612 (0~100 um)" class="Clust"("Value"=w849) -> ()  [unwired: 2 in, 2 out]
              }
            }
          }
          frame "Y" {
            n439 = flat-sequence {
              tunnel: w863 -> [w867]
              tunnel: [w869] -> w862
              tunnel: [w868] -> w861
              tunnel: [w867] -> w860
              tunnel: w859 -> [w866]
              tunnel: w858 -> [w865]
              tunnel: w862 -> [w878]
              tunnel: w861 -> [w877]
              tunnel: w860 -> [w876]
              frame #0 {
                w868 = bool[] [TRUE, TRUE] ("Axis")
                n440 = control-ref of="Abort AllStage"() -> (w869:refnum<vi>)
                n441 = Build Array(w866, w865) -> (w864:dbl[])
                n442 = call "AE_AllStages_Action V2.vi"("Velocity"=3.0, "Abort"=w869, "Positions"=w864, "Axis"=w868, "Stage ID"="P612", "Action"=StageStates."MOVE") -> ()  [unwired: 3 in, 3 out]
              }
              frame #1 {
                w880 = FALSE
                n443 = call "AE_AllStages_Action V2.vi"("Abort"=w878, "Axis"=w877, "Stage ID"="P612", "Action"=StageStates."POSITION") -> ("Position Out"=w881:dbl[])  [unwired: 5 in, 2 out]
                n444 = Index Array(array=w881, index #1=0 ("index"), index #2=1 ("index")) -> (element #1=w879:dbl, element #2=w873:dbl)
                n445 = Bundle(w880, w880, w880, w880, w880, "Step Size (um)"=w876, "Numeric"=w879, "Numeric"=w873) -> (w875:T31)  [unwired: 1 in]
                n446 = property on="Bottom Objective Holder XY - P612 (0~100 um)" class="Clust"("Value"=w875) -> ()  [unwired: 2 in, 2 out]
              }
            }
          }
          frame "Step Size (um)" {
            w888 = FALSE
            n447 = control-ref of="Abort AllStage"() -> (w896:refnum<vi>)
            n448 = call "AE_AllStages_Action V2.vi"("Abort"=w896, "Axis"=bool[] [TRUE, TRUE], "Stage ID"="P612", "Action"=StageStates."POSITION") -> ("Position Out"=w890:dbl[])  [unwired: 5 in, 2 out]
            n449 = Index Array(array=w890, index=0) -> (element=w887:dbl)
            n450 = Index Array(array=w890, index=1) -> (element=w886:dbl)
            n451 = Bundle(w888, w888, w888, w888, w888, "Step Size (um)"=w894, "Numeric"=w887, "Numeric"=w886) -> (w885:T31)  [unwired: 1 in]
            n452 = property on="Bottom Objective Holder XY - P612 (0~100 um)" class="Clust"("Value"=w885) -> ()  [unwired: 2 in, 2 out]
          }
        }
      }
      event "Radio Buttons": Value Change {
        n453 = event-data() -> ()  [unwired: 1 in, 6 out]
        n454 = case shown="\"Radio Selection 2\"" "Radio Buttons" {
          frame "Radio Selection 1", Default {
            n455 = property on="Joystick Velocity" class="CmbBox"("DisabledEnum"=T19."Enabled" ("Disabled")) -> ()  [unwired: 2 in, 2 out]
            n456 = property on="Sample Stage XY - M686" class="Clust"("DisabledEnum"=T19."Disabled and Grayed Out" ("Disabled")) -> ()  [unwired: 2 in, 2 out]
          }
          frame "Radio Selection 2" {
            n457 = Unbundle By Name("Sample Stage XY - M686") -> ("Step Size (um)"=w905:dbl, "X"=w904:dbl, "Y"=w903:dbl)
            n458 = event shown="[1] \"Sample Stage XY - M686.Home Button\", \"Sample Stage XY - M686.Up Button\", \"Sample Stage XY - M686.Left Button\", \"Sample Stage XY - M686.Down Button\", \"Sample Stage XY - M686.Right Button\", \"Sample Stage XY - M686.Step Size (um)\", \"Sample Stage XY - M686.X\", \"Sample Stage XY - M686.Y\": Value Change" {
              selector: _ -> [_ _]
              dyn-events: _ -> [_ _]
              timeout: 30 -> [_ _]
              tunnel: w905 -> [_ w908]
              tunnel: w904 -> [_ w912]
              tunnel: w903 -> [_ w911]
              tunnel: "Sample Stage XY - M686" -> [_ w909]
              event Timeout {
                n459 = event-data() -> ()  [unwired: 1 in, 3 out]
              }
              event Value Change {
                n460 = event-data() -> ("CtlRef"=w919:refnum<vi>)  [unwired: 1 in, 2 out]
                n461 = control-ref of="Abort AllStage"() -> (w915:refnum<vi>)
                n462 = property class="Ctl"(reference=w919) -> ("Label.Text"=w918:string)  [unwired: 1 in, 2 out]
                n463 = Build Array(w912, w911) -> (w910:dbl[])
                n464 = Divide(x=w908, y=1000.0) -> (x/y=w914:dbl)
                n465 = case shown="\"X\"" w918 {
                  tunnel: "M686" ("Stage ID") -> [w923 w949 w977 w1007 w1036 w1066 w1080 w1107]
                  tunnel: bool[] [TRUE, FALSE] ("Axis") -> [w922 w948 w976 w1006 w1035 w1071 w1079 w1106]
                  tunnel: w915 -> [w925 w951 w979 w1009 w1038 w1065 w1073 w1102]
                  tunnel: w914 -> [_ w946 w974 w1004 w1033 _ w1075 _]
                  tunnel: w910 -> [_ _ _ _ _ _ w1078 w1105]
                  tunnel: w909 -> [_ _ _ _ _ _ w1072 _]
                  tunnel: w908 -> [w920 w945 w973 w1003 w1032 w1060 _ w1101]
                  frame "Home Button", Default {
                    n466 = flat-sequence {
                      tunnel: w925 -> [w930]
                      tunnel: [w928] -> w924
                      tunnel: w923 -> [w929]
                      tunnel: w922 -> [w928]
                      tunnel: [w926] -> w921
                      tunnel: w920 -> [w926]
                      tunnel: w925 -> [w936]
                      tunnel: w924 -> [w935]
                      tunnel: w921 -> [w934]
                      frame #0 {
                        n467 = call "AE_AllStages_Action V2.vi"("Velocity"=10.0, "Abort"=w930, "Positions"=dbl[] [12.5, 12.5], "Axis"=w928, "Stage ID"=w929, "Action"=StageStates."MOVE") -> ()  [unwired: 3 in, 3 out]
                      }
                      frame #1 {
                        w941 = FALSE
                        n468 = call "AE_AllStages_Action V2.vi"("Abort"=w936, "Axis"=w935, "Stage ID"="M686", "Action"=StageStates."POSITION") -> ("Position Out"=w939:dbl[])  [unwired: 5 in, 2 out]
                        n469 = Index Array(array=w939, index=0) -> (element=w942:dbl)
                        n470 = Index Array(array=w939, index=1) -> (element=w943:dbl)
                        n471 = Bundle(w941, w941, w941, w941, w941, "Step Size (um)"=w934, "Numeric"=w942, "Numeric"=w943) -> (w944:T31)  [unwired: 1 in]
                        n472 = property on="Sample Stage XY - M686" class="Clust"("Value"=w944) -> ()  [unwired: 2 in, 2 out]
                      }
                    }
                  }
                  frame "Left Button" {
                    n473 = flat-sequence {
                      tunnel: w951 -> [w959]
                      tunnel: [w957] -> w950
                      tunnel: w949 -> [w958]
                      tunnel: w948 -> [w957]
                      tunnel: [w952] -> w947
                      tunnel: w946 -> [w956]
                      tunnel: w945 -> [w952]
                      tunnel: w951 -> [w964]
                      tunnel: w950 -> [w963]
                      tunnel: w947 -> [w962]
                      frame #0 {
                        n474 = Build Array(w956, 0.0 ("element")) -> (w955:dbl[])
                        n475 = call "AE_AllStages_Action V2.vi"("Velocity"=10.0, "Abort"=w959, "Positions"=w955, "Axis"=w957, "Stage ID"=w958, "Action"=StageStates."MVR") -> ()  [unwired: 3 in, 3 out]
                      }
                      frame #1 {
                        w969 = FALSE
                        n476 = call "AE_AllStages_Action V2.vi"("Abort"=w964, "Axis"=w963, "Stage ID"="M686", "Action"=StageStates."POSITION") -> ("Position Out"=w967:dbl[])  [unwired: 5 in, 2 out]
                        n477 = Index Array(array=w967, index=0) -> (element=w970:dbl)
                        n478 = Index Array(array=w967, index=1) -> (element=w971:dbl)
                        n479 = Bundle(w969, w969, w969, w969, w969, "Step Size (um)"=w962, "Numeric"=w970, "Numeric"=w971) -> (w972:T31)  [unwired: 1 in]
                        n480 = property on="Sample Stage XY - M686" class="Clust"("Value"=w972) -> ()  [unwired: 2 in, 2 out]
                      }
                    }
                  }
                  frame "Right Button" {
                    n481 = flat-sequence {
                      tunnel: w979 -> [w989]
                      tunnel: [w987] -> w978
                      tunnel: w977 -> [w988]
                      tunnel: w976 -> [w987]
                      tunnel: [w980] -> w975
                      tunnel: w974 -> [w983]
                      tunnel: w973 -> [w980]
                      tunnel: w979 -> [w994]
                      tunnel: w978 -> [w993]
                      tunnel: w975 -> [w992]
                      frame #0 {
                        n482 = Subtract(x=0.0, y=w983) -> (x-y=w984:dbl)
                        n483 = Build Array(w984, 0.0 ("element")) -> (w986:dbl[])
                        n484 = call "AE_AllStages_Action V2.vi"("Velocity"=10.0, "Abort"=w989, "Positions"=w986, "Axis"=w987, "Stage ID"=w988, "Action"=StageStates."MVR") -> ()  [unwired: 3 in, 3 out]
                      }
                      frame #1 {
                        w999 = FALSE
                        n485 = call "AE_AllStages_Action V2.vi"("Abort"=w994, "Axis"=w993, "Stage ID"="M686", "Action"=StageStates."POSITION") -> ("Position Out"=w997:dbl[])  [unwired: 5 in, 2 out]
                        n486 = Index Array(array=w997, index=0) -> (element=w1000:dbl)
                        n487 = Index Array(array=w997, index=1) -> (element=w1001:dbl)
                        n488 = Bundle(w999, w999, w999, w999, w999, "Step Size (um)"=w992, "Numeric"=w1000, "Numeric"=w1001) -> (w1002:T31)  [unwired: 1 in]
                        n489 = property on="Sample Stage XY - M686" class="Clust"("Value"=w1002) -> ()  [unwired: 2 in, 2 out]
                      }
                    }
                  }
                  frame "Up Button" {
                    n490 = flat-sequence {
                      tunnel: w1009 -> [w1018]
                      tunnel: [w1016] -> w1008
                      tunnel: w1007 -> [w1017]
                      tunnel: w1006 -> [w1016]
                      tunnel: [w1010] -> w1005
                      tunnel: w1004 -> [w1013]
                      tunnel: w1003 -> [w1010]
                      tunnel: w1009 -> [w1023]
                      tunnel: w1008 -> [w1022]
                      tunnel: w1005 -> [w1021]
                      frame #0 {
                        w1012 = 0.0 ("x")
                        n491 = Subtract(x=w1012, y=w1013) -> (x-y=w1014:dbl)
                        n492 = Build Array(w1012, w1014) -> (w1015:dbl[])
                        n493 = call "AE_AllStages_Action V2.vi"("Velocity"=10.0, "Abort"=w1018, "Positions"=w1015, "Axis"=w1016, "Stage ID"=w1017, "Action"=StageStates."MVR") -> ()  [unwired: 3 in, 3 out]
                      }
                      frame #1 {
                        w1028 = FALSE
                        n494 = call "AE_AllStages_Action V2.vi"("Abort"=w1023, "Axis"=w1022, "Stage ID"="M686", "Action"=StageStates."POSITION") -> ("Position Out"=w1026:dbl[])  [unwired: 5 in, 2 out]
                        n495 = Index Array(array=w1026, index=0) -> (element=w1029:dbl)
                        n496 = Index Array(array=w1026, index=1) -> (element=w1030:dbl)
                        n497 = Bundle(w1028, w1028, w1028, w1028, w1028, "Step Size (um)"=w1021, "Numeric"=w1029, "Numeric"=w1030) -> (w1031:T31)  [unwired: 1 in]
                        n498 = property on="Sample Stage XY - M686" class="Clust"("Value"=w1031) -> ()  [unwired: 2 in, 2 out]
                      }
                    }
                  }
                  frame "Down Button" {
                    n499 = flat-sequence {
                      tunnel: w1038 -> [w1046]
                      tunnel: [w1044] -> w1037
                      tunnel: w1036 -> [w1045]
                      tunnel: w1035 -> [w1044]
                      tunnel: [w1039] -> w1034
                      tunnel: w1033 -> [w1041]
                      tunnel: w1032 -> [w1039]
                      tunnel: w1038 -> [w1051]
                      tunnel: w1037 -> [w1050]
                      tunnel: w1034 -> [w1049]
                      frame #0 {
                        n500 = Build Array(0.0 ("x"), w1041) -> (w1043:dbl[])
                        n501 = call "AE_AllStages_Action V2.vi"("Velocity"=10.0, "Abort"=w1046, "Positions"=w1043, "Axis"=w1044, "Stage ID"=w1045, "Action"=StageStates."MVR") -> ()  [unwired: 3 in, 3 out]
                      }
                      frame #1 {
                        w1056 = FALSE
                        n502 = call "AE_AllStages_Action V2.vi"("Abort"=w1051, "Axis"=w1050, "Stage ID"="M686", "Action"=StageStates."POSITION") -> ("Position Out"=w1054:dbl[])  [unwired: 5 in, 2 out]
                        n503 = Index Array(array=w1054, index=0) -> (element=w1057:dbl)
                        n504 = Index Array(array=w1054, index=1) -> (element=w1058:dbl)
                        n505 = Bundle(w1056, w1056, w1056, w1056, w1056, "Step Size (um)"=w1049, "Numeric"=w1057, "Numeric"=w1058) -> (w1059:T31)  [unwired: 1 in]
                        n506 = property on="Sample Stage XY - M686" class="Clust"("Value"=w1059) -> ()  [unwired: 2 in, 2 out]
                      }
                    }
                  }
                  frame "Step Size (um)" {
                    w1061 = FALSE
                    n507 = call "AE_AllStages_Action V2.vi"("Abort"=w1065, "Axis"=w1071, "Stage ID"=w1066, "Action"=StageStates."POSITION") -> ("Position Out"=w1069:dbl[])  [unwired: 5 in, 2 out]
                    n508 = Index Array(array=w1069, index=0) -> (element=w1063:dbl)
                    n509 = Index Array(array=w1069, index=1) -> (element=w1062:dbl)
                    n510 = Bundle(w1061, w1061, w1061, w1061, w1061, "Step Size (um)"=w1060, "Numeric"=w1063, "Numeric"=w1062) -> (w1064:T31)  [unwired: 1 in]
                    n511 = property on="Sample Stage XY - M686" class="Clust"("Value"=w1064) -> ()  [unwired: 2 in, 2 out]
                  }
                  frame "X" {
                    n512 = flat-sequence {
                      tunnel: w1073 -> [w1087]
                      tunnel: w1080 -> [w1083]
                      tunnel: w1079 -> [w1084]
                      tunnel: w1078 -> [w1085]
                      tunnel: [w1084] -> w1077
                      tunnel: [w1083] -> w1076
                      tunnel: w1075 -> [w1082]
                      tunnel: [w1082] -> w1074
                      tunnel: w1077 -> [w1095]
                      tunnel: w1076 -> [w1094]
                      tunnel: w1074 -> [_]
                      tunnel: w1073 -> [w1093]
                      tunnel: w1072 -> [w1092]
                      frame #0 {
                        n513 = call "AE_AllStages_Action V2.vi"("Velocity"=10.0, "Abort"=w1087, "Positions"=w1085, "Axis"=w1084, "Stage ID"=w1083, "Action"=StageStates."MOVE") -> ()  [unwired: 3 in, 3 out]
                      }
                      frame #1 {
                        w1091 = FALSE
                        n514 = call "AE_AllStages_Action V2.vi"("Abort"=w1093, "Axis"=w1095, "Stage ID"=w1094, "Action"=StageStates."POSITION") -> ("Position Out"=w1097:dbl[])  [unwired: 5 in, 2 out]
                        n515 = Index Array(array=w1097, index=0) -> (element=w1090:dbl)
                        n516 = Index Array(array=w1097, index=1) -> (element=w1089:dbl)
                        n517 = Bundle By Name(cluster=w1092, "Home Button"=w1091, "Up Button"=w1091, "Left Button"=w1091, "Down Button"=w1091, "Right Button"=w1091, "X"=w1090, "Y"=w1089) -> (w1088:T3)
                        n518 = property on="Sample Stage XY - M686" class="Clust"("Value"=w1088) -> ()  [unwired: 2 in, 2 out]
                      }
                    }
                  }
                  frame "Y" {
                    n519 = flat-sequence {
                      tunnel: w1102 -> [w1114]
                      tunnel: w1107 -> [w1110]
                      tunnel: w1106 -> [w1111]
                      tunnel: w1105 -> [w1112]
                      tunnel: [w1111] -> w1104
                      tunnel: [w1110] -> w1103
                      tunnel: w1101 -> [w1108]
                      tunnel: [w1108] -> w1100
                      tunnel: w1104 -> [w1119]
                      tunnel: w1103 -> [w1118]
                      tunnel: w1102 -> [w1116]
                      tunnel: w1100 -> [w1115]
                      frame #0 {
                        n520 = call "AE_AllStages_Action V2.vi"("Velocity"=10.0, "Abort"=w1114, "Positions"=w1112, "Axis"=w1111, "Stage ID"=w1110, "Action"=StageStates."MOVE") -> ()  [unwired: 3 in, 3 out]
                      }
                      frame #1 {
                        w1122 = FALSE
                        n521 = call "AE_AllStages_Action V2.vi"("Abort"=w1116, "Axis"=w1119, "Stage ID"=w1118, "Action"=StageStates."POSITION") -> ("Position Out"=w1124:dbl[])  [unwired: 5 in, 2 out]
                        n522 = Index Array(array=w1124, index=0) -> (element=w1121:dbl)
                        n523 = Index Array(array=w1124, index=1) -> (element=w1120:dbl)
                        n524 = Bundle(w1122, w1122, w1122, w1122, w1122, "Step Size (um)"=w1115, "Numeric"=w1121, "Numeric"=w1120) -> (w1117:T31)  [unwired: 1 in]
                        n525 = property on="Sample Stage XY - M686" class="Clust"("Value"=w1117) -> ()  [unwired: 2 in, 2 out]
                      }
                    }
                  }
                }
              }
            }
            n526 = property on="Joystick Velocity" class="CmbBox"("DisabledEnum"=T19."Disabled and Grayed Out" ("Disabled")) -> ()  [unwired: 2 in, 2 out]
            n527 = property on="Sample Stage XY - M686" class="Clust"("DisabledEnum"=T19."Enabled" ("Disabled")) -> ()  [unwired: 2 in, 2 out]
          }
        }
      }
      event Value Change {
        n528 = event-data() -> ("NewVal"=w1130:dbl)  [unwired: 1 in]
        n529 = flat-sequence {
          tunnel: w1130 -> [w1137]
          tunnel: [w1131] -> w1129
          tunnel: w1129 -> [w1143]
          tunnel: "Phase Compensation Mirror - P841 (0~15 um)" -> [w1140]
          frame #0 {
            n530 = control-ref of="Abort AllStage"() -> (w1131:refnum<vi>)
            n531 = Build Array(w1137) -> (w1136:dbl[])
            n532 = call "AE_AllStages_Action V2.vi"("Velocity"=10000.0, "Abort"=w1131, "Positions"=w1136, "Axis"=bool[] [TRUE], "Stage ID"="P841", "Action"=StageStates."MOVE") -> ()  [unwired: 3 in, 3 out]
          }
          frame #1 {
            n533 = call "AE_AllStages_Action V2.vi"("Abort"=w1143, "Axis"=bool[] [TRUE], "Stage ID"="P841", "Action"=StageStates."POSITION") -> ("Position Out"=w1142:dbl[])  [unwired: 5 in, 2 out]
            n534 = Index Array(array=w1142, index=0) -> (element=w1139:dbl)
            n535 = Bundle By Name(cluster=w1140, "Position (µm)"=w1139) -> (w1138:T2)
            n536 = property on="Phase Compensation Mirror - P841 (0~15 um)" class="Clust"("Value"=w1138) -> ()  [unwired: 2 in, 2 out]
          }
        }
      }
      event Value Change {
        n537 = event-data() -> ("CtlRef"=w1155:refnum<vi>)  [unwired: 1 in, 2 out]
        n538 = property class="Ctl"(reference=w1155) -> ("Label.Text"=w1154:string)  [unwired: 1 in, 2 out]
        n539 = Unbundle By Name("4Pi Cavity Translation Z - ASI") -> ("Velocity"=w1148:dbl, "Step Size (um)"=w1153:dbl, "Position (mm)"=w1152:dbl, "Z (um)"=w1151:dbl, "F (um)"=w1150:dbl)
        n540 = case shown="\"Step Size (um)\"" w1154 {
          tunnel: w1153 -> [w1158 w1195 w1237 w1268 w1301 w1328]
          tunnel: w1152 -> [_ _ _ _ w1296 _]
          tunnel: w1151 -> [w1160 w1197 w1233 _ _ _]
          tunnel: w1150 -> [w1159 w1196 _ w1264 _ _]
          tunnel: w1148 -> [w1157 w1194 w1232 w1263 w1294 w1326]
          frame "Down Button" {
            n541 = flat-sequence {
              tunnel: w1158 -> [w1169]
              tunnel: [w1174] -> w1161
              tunnel: w1160 -> [w1171]
              tunnel: w1159 -> [w1170]
              tunnel: w1157 -> [w1162]
              tunnel: [w1162] -> w1156
              tunnel: w1161 -> [w1189]
              tunnel: w1158 -> [w1178]
              tunnel: w1156 -> [w1177]
              frame #0 {
                n542 = Multiply(x=2.0, y=w1169) -> (x*y=w1167:dbl)
                n543 = Add(x=w1171, y=w1170) -> (x+y=w1166:dbl)
                n544 = Add(x=w1167, y=w1166) -> (x+y=w1165:dbl)
                n545 = Divide(x=w1165, y=2.0) -> (x/y=w1163:dbl)
                n546 = control-ref of="Abort AllStage"() -> (w1174:refnum<vi>)
                n547 = Build Array(w1163, w1163) -> (w1172:dbl[])
                n548 = call "AE_AllStages_Action V2.vi"("Velocity"=w1162, "Abort"=w1174, "Positions"=w1172, "Axis"=bool[] [TRUE, TRUE], "Stage ID"="ASI", "Action"=StageStates."MOVE") -> ()  [unwired: 3 in, 3 out]
              }
              frame #1 {
                w1183 = FALSE
                n549 = call "AE_AllStages_Action V2.vi"("Abort"=w1189, "Axis"=bool[] [TRUE, TRUE], "Stage ID"="ASI", "Action"=StageStates."POSITION") -> ("Position Out"=w1182:dbl[])  [unwired: 5 in, 2 out]
                n550 = Add Array Elements(numeric array=w1182) -> (sum=w1181:dbl)
                n551 = Index Array(array=w1182, index #1=0 ("index"), index #2=1 ("index")) -> (element #1=w1185:dbl, element #2=w1184:dbl)
                n552 = Divide(x=w1181, y=2000.0) -> (x/y=w1179:dbl)
                n553 = Bundle(w1183, w1183, "Step Size (um)"=w1178, w1179, "Numeric"=w1185, "Numeric"=w1184, "Velocity"=w1177) -> (w1186:T32)  [unwired: 1 in]
                n554 = property on="4Pi Cavity Translation Z - ASI" class="Clust"("Value"=w1186) -> ()  [unwired: 2 in, 2 out]
              }
            }
          }
          frame "Up Button" {
            n555 = flat-sequence {
              tunnel: w1195 -> [w1207]
              tunnel: [w1212] -> w1198
              tunnel: w1197 -> [w1209]
              tunnel: w1196 -> [w1208]
              tunnel: w1194 -> [w1200]
              tunnel: [w1200] -> w1193
              tunnel: w1198 -> [w1227]
              tunnel: w1195 -> [w1216]
              tunnel: w1193 -> [w1215]
              frame #0 {
                n556 = Multiply(x=2.0, y=w1207) -> (x*y=w1202:dbl)
                n557 = Add(x=w1209, y=w1208) -> (x+y=w1201:dbl)
                n558 = Subtract(x=w1201, y=w1202) -> (x-y=w1205:dbl)
                n559 = Divide(x=w1205, y=2.0) -> (x/y=w1203:dbl)
                n560 = control-ref of="Abort AllStage"() -> (w1212:refnum<vi>)
                n561 = Build Array(w1203, w1203) -> (w1210:dbl[])
                n562 = call "AE_AllStages_Action V2.vi"("Velocity"=w1200, "Abort"=w1212, "Positions"=w1210, "Axis"=bool[] [TRUE, TRUE], "Stage ID"="ASI", "Action"=StageStates."MOVE") -> ()  [unwired: 3 in, 3 out]
                n563 = local write "ASI"(TRUE ("Moving")) -> ()
              }
              frame #1 {
                w1221 = FALSE
                n564 = call "AE_AllStages_Action V2.vi"("Abort"=w1227, "Axis"=bool[] [TRUE, TRUE], "Stage ID"="ASI", "Action"=StageStates."POSITION") -> ("Position Out"=w1220:dbl[])  [unwired: 5 in, 2 out]
                n565 = Add Array Elements(numeric array=w1220) -> (sum=w1219:dbl)
                n566 = Index Array(array=w1220, index #1=0 ("index"), index #2=1 ("index")) -> (element #1=w1223:dbl, element #2=w1222:dbl)
                n567 = Divide(x=w1219, y=2000.0) -> (x/y=w1217:dbl)
                n568 = Bundle(w1221, w1221, "Step Size (um)"=w1216, w1217, "Numeric"=w1223, "Numeric"=w1222, "Velocity"=w1215) -> (w1224:T32)  [unwired: 1 in]
                n569 = property on="4Pi Cavity Translation Z - ASI" class="Clust"("Value"=w1224) -> ()  [unwired: 2 in, 2 out]
              }
            }
          }
          frame "Z (um)" {
            n570 = flat-sequence {
              tunnel: w1237 -> [w1241]
              tunnel: [w1243] -> w1236
              tunnel: [w1242] -> w1235
              tunnel: [w1241] -> w1234
              tunnel: w1233 -> [w1239]
              tunnel: w1232 -> [w1238]
              tunnel: [w1238] -> w1231
              tunnel: w1236 -> [w1259]
              tunnel: w1235 -> [w1258]
              tunnel: w1234 -> [w1248]
              tunnel: w1231 -> [w1246]
              frame #0 {
                w1242 = bool[] [TRUE, TRUE] ("Axis")
                n571 = control-ref of="Abort AllStage"() -> (w1243:refnum<vi>)
                n572 = Build Array(w1239, w1239) -> (w1240:dbl[])
                n573 = call "AE_AllStages_Action V2.vi"("Velocity"=w1238, "Abort"=w1243, "Positions"=w1240, "Axis"=w1242, "Stage ID"="ASI", "Action"=StageStates."MOVE") -> ()  [unwired: 3 in, 3 out]
              }
              frame #1 {
                w1252 = FALSE
                n574 = call "AE_AllStages_Action V2.vi"("Abort"=w1259, "Axis"=w1258, "Stage ID"="ASI", "Action"=StageStates."POSITION") -> ("Position Out"=w1247:dbl[])  [unwired: 5 in, 2 out]
                n575 = Add Array Elements(numeric array=w1247) -> (sum=w1251:dbl)
                n576 = Index Array(array=w1247, index #1=0 ("index"), index #2=1 ("index")) -> (element #1=w1254:dbl, element #2=w1253:dbl)
                n577 = Divide(x=w1251, y=2000.0) -> (x/y=w1249:dbl)
                n578 = Bundle(w1252, w1252, "Step Size (um)"=w1248, w1249, "Numeric"=w1254, "Numeric"=w1253, "Velocity"=w1246) -> (w1255:T32)  [unwired: 1 in]
                n579 = property on="4Pi Cavity Translation Z - ASI" class="Clust"("Value"=w1255) -> ()  [unwired: 2 in, 2 out]
              }
            }
          }
          frame "F (um)" {
            n580 = flat-sequence {
              tunnel: w1268 -> [w1272]
              tunnel: [w1274] -> w1267
              tunnel: [w1273] -> w1266
              tunnel: [w1272] -> w1265
              tunnel: w1264 -> [w1270]
              tunnel: w1263 -> [w1269]
              tunnel: [w1269] -> w1262
              tunnel: w1267 -> [w1290]
              tunnel: w1266 -> [w1289]
              tunnel: w1265 -> [w1279]
              tunnel: w1262 -> [w1277]
              frame #0 {
                w1273 = bool[] [TRUE, TRUE] ("Axis")
                n581 = control-ref of="Abort AllStage"() -> (w1274:refnum<vi>)
                n582 = Build Array(w1270, w1270) -> (w1271:dbl[])
                n583 = call "AE_AllStages_Action V2.vi"("Velocity"=w1269, "Abort"=w1274, "Positions"=w1271, "Axis"=w1273, "Stage ID"="ASI", "Action"=StageStates."MOVE") -> ()  [unwired: 3 in, 3 out]
              }
              frame #1 {
                w1283 = FALSE
                n584 = call "AE_AllStages_Action V2.vi"("Abort"=w1290, "Axis"=w1289, "Stage ID"="ASI", "Action"=StageStates."POSITION") -> ("Position Out"=w1278:dbl[])  [unwired: 5 in, 2 out]
                n585 = Add Array Elements(numeric array=w1278) -> (sum=w1282:dbl)
                n586 = Index Array(array=w1278, index #1=0 ("index"), index #2=1 ("index")) -> (element #1=w1285:dbl, element #2=w1284:dbl)
                n587 = Divide(x=w1282, y=2000.0) -> (x/y=w1280:dbl)
                n588 = Bundle(w1283, w1283, "Step Size (um)"=w1279, w1280, "Numeric"=w1285, "Numeric"=w1284, "Velocity"=w1277) -> (w1286:T32)  [unwired: 1 in]
                n589 = property on="4Pi Cavity Translation Z - ASI" class="Clust"("Value"=w1286) -> ()  [unwired: 2 in, 2 out]
              }
            }
          }
          frame "Position (mm)", Default {
            n590 = Multiply(x=w1296, y=1000.0) -> (x*y=w1297:dbl)
            n591 = flat-sequence {
              tunnel: w1301 -> [w1305]
              tunnel: [w1307] -> w1300
              tunnel: [w1306] -> w1299
              tunnel: [w1305] -> w1298
              tunnel: w1297 -> [w1303]
              tunnel: w1294 -> [w1302]
              tunnel: [w1302] -> w1293
              tunnel: w1300 -> [w1323]
              tunnel: w1299 -> [w1322]
              tunnel: w1298 -> [w1312]
              tunnel: w1293 -> [w1310]
              frame #0 {
                w1306 = bool[] [TRUE, TRUE] ("Axis")
                n592 = control-ref of="Abort AllStage"() -> (w1307:refnum<vi>)
                n593 = Build Array(w1303, w1303) -> (w1304:dbl[])
                n594 = call "AE_AllStages_Action V2.vi"("Velocity"=w1302, "Abort"=w1307, "Positions"=w1304, "Axis"=w1306, "Stage ID"="ASI", "Action"=StageStates."MOVE") -> ()  [unwired: 3 in, 3 out]
              }
              frame #1 {
                w1316 = FALSE
                n595 = call "AE_AllStages_Action V2.vi"("Abort"=w1323, "Axis"=w1322, "Stage ID"="ASI", "Action"=StageStates."POSITION") -> ("Position Out"=w1311:dbl[])  [unwired: 5 in, 2 out]
                n596 = Add Array Elements(numeric array=w1311) -> (sum=w1315:dbl)
                n597 = Index Array(array=w1311, index #1=0 ("index"), index #2=1 ("index")) -> (element #1=w1318:dbl, element #2=w1317:dbl)
                n598 = Divide(x=w1315, y=2000.0) -> (x/y=w1313:dbl)
                n599 = Bundle(w1316, w1316, "Step Size (um)"=w1312, w1313, "Numeric"=w1318, "Numeric"=w1317, "Velocity"=w1310) -> (w1319:T32)  [unwired: 1 in]
                n600 = property on="4Pi Cavity Translation Z - ASI" class="Clust"("Value"=w1319) -> ()  [unwired: 2 in, 2 out]
              }
            }
          }
          frame "Step Size (um)" {
            w1332 = FALSE
            n601 = control-ref of="Abort AllStage"() -> (w1341:refnum<vi>)
            n602 = call "AE_AllStages_Action V2.vi"("Abort"=w1341, "Axis"=bool[] [TRUE, TRUE], "Stage ID"="ASI", "Action"=StageStates."POSITION") -> ("Position Out"=w1327:dbl[])  [unwired: 5 in, 2 out]
            n603 = Add Array Elements(numeric array=w1327) -> (sum=w1331:dbl)
            n604 = Index Array(array=w1327, index #1=0 ("index"), index #2=1 ("index")) -> (element #1=w1334:dbl, element #2=w1333:dbl)
            n605 = Divide(x=w1331, y=2000.0) -> (x/y=w1329:dbl)
            n606 = Bundle(w1332, w1332, "Step Size (um)"=w1328, w1329, "Numeric"=w1334, "Numeric"=w1333, "Velocity"=w1326) -> (w1335:T32)  [unwired: 1 in]
            n607 = property on="4Pi Cavity Translation Z - ASI" class="Clust"("Value"=w1335) -> ()  [unwired: 2 in, 2 out]
          }
        }
      }
      event "Upper Shutter", "Lower Shutter": Value Change {
        n608 = event-data() -> ()  [unwired: 1 in, 1 out]
        n609 = Not(x="Upper Shutter") -> (.not. x?=w1346:bool)
        n610 = Not(x="Lower Shutter") -> (.not. x?=w1345:bool)
        n611 = Bundle(w1346, w1345) -> (w1348:cluster{bool, bool})  [unwired: 1 in]
        n612 = call "FPGA-7842R-Control V1.vi"(1:w1348, "Action"=FPGA-7842R-Reference."Shutter Control", "Initialize"=TRUE) -> ()  [unwired: 11 in, 2 out]
      }
      event "Load Positions": Value Change {
        n613 = event-data() -> ()  [unwired: 1 in, 6 out]
        n614 = call "Load Stage Positions.vi"() -> ("appended array"=w1362:bool[])  [unwired: 1 in]
        n615 = control-ref of="Abort AllStage"() -> (w1360:refnum<vi>)
        n616 = Build Array("P841", "M686", "M686", "P612") -> (w1361:string[])
        n617 = TDMS Open(10:T24."open (read-only)" ("operation (0:open)"), 11:path "C:/Users/ED STED/Documents/Test Control Software/Host VIs/Stages/Stage Positions/Stage Positions in Last Experiment.tdms" ("file path")) -> (3:w1356:refnum<k34>)  [unwired: 5 in, 1 out]
        n618 = TDMS Read(0:w1356, 5:"Stage Positions" ("group name in (Untitled)")) -> (4:w1355:refnum<k34>, 10:w1353:waveform(dbl)[])  [unwired: 6 in, 4 out]
        n619 = Index Array(array=w1353, index=0) -> (element=w1351:waveform(dbl))
        n620 = TDMS Close(11:w1355) -> ()  [unwired: 1 in, 2 out]
        n621 = Unbundle By Name(w1351) -> ("Y"=w1350:dbl[])
        n622 = for {
          N -> [w1368]
          tunnel: w1362 -> [w1371] mode=indexing
          tunnel: w1361 -> [w1370] mode=indexing
          tunnel: w1360 -> [w1369]
          tunnel: w1350 -> [w1367] mode=indexing
          n623 = case shown="True" w1371 {
            tunnel: w1370 -> [_ w1374]
            tunnel: w1369 -> [_ w1375]
            tunnel: w1368 -> [_ w1373]
            tunnel: w1367 -> [_ w1372]
            frame False {
            }
            frame True {
              n624 = case shown="\"P612\", Default" w1374 {
                tunnel: w1375 -> [w1379 w1404 w1432]
                tunnel: w1374 -> [w1380 w1405 w1433]
                tunnel: w1373 -> [_ w1401 w1429]
                tunnel: w1372 -> [w1377 w1400 w1428]
                frame "P612", Default {
                  n625 = flat-sequence {
                    tunnel: w1380 -> [w1391]
                    tunnel: w1379 -> [w1392]
                    tunnel: [w1392] -> w1378
                    tunnel: w1377 -> [w1381]
                    tunnel: [w1391] -> w1376
                    tunnel: w1378 -> [w1398]
                    tunnel: w1376 -> [w1394]
                    frame #0 {
                      n626 = Divide(x=w1381, y=10.0) -> (x/y=w1384:dbl)
                      n627 = call "Volts to I16.vi"("Voltage (V)"=w1384) -> ("I16"=w1385:i16)  [unwired: 13 in, 1 out]
                      n628 = call "Manual Controls Action Engine.vi"("Action"=enum16{"Read", "Write"}."Read") -> ("Manual Controls Out"=w1386:T18)  [unwired: 14 in]
                      n629 = Bundle By Name(cluster=w1386, "Z Axis Voltage (I16)"=w1385) -> (w1389:T18)
                      n630 = call "Manual Controls Action Engine.vi"("Action"=enum16{"Read", "Write"}."Write", "Manual Controls In"=w1389) -> ()  [unwired: 13 in, 1 out]
                      n631 = call "FPGA-7842R-Control V1.vi"("Action"=FPGA-7842R-Reference."Stage Control", "Manual Controls"=w1389, "Initialize"=TRUE) -> ()  [unwired: 11 in, 2 out]
                    }
                    frame #1 {
                      n632 = call "AE_AllStages_Action V2.vi"("Abort"=w1398, "Axis"=bool[] [TRUE, TRUE, TRUE], "Stage ID"=w1394, "Action"=StageStates."POSITION") -> ("Position Out"=w1397:dbl[])  [unwired: 5 in, 2 out]
                      n633 = Index Array(array=w1397, index=2) -> (element=w1395:dbl)
                    }
                  }
                }
                frame "M686" {
                  n634 = flat-sequence {
                    tunnel: w1405 -> [w1417]
                    tunnel: w1404 -> [w1412]
                    tunnel: [w1412] -> w1403
                    tunnel: [w1410] -> w1402
                    tunnel: w1401 -> [w1409]
                    tunnel: w1400 -> [w1406]
                    tunnel: w1403 -> [w1426]
                    tunnel: w1402 -> [w1424]
                    frame #0 {
                      w1410 = bool[] [TRUE, TRUE] ("Axis")
                      n635 = call "AE_AllStages_Action V2.vi"("Abort"=w1412, "Axis"=w1410, "Stage ID"=w1417, "Action"=StageStates."POSITION") -> ("Position Out"=w1416:dbl[])  [unwired: 5 in, 2 out]
                      n636 = Subtract(x=w1409, y=1) -> (x-y=w1407:i32)
                      n637 = Replace Array Subset(array=w1416, new element=w1406, index=w1407) -> (w1415:dbl[])
                      n638 = call "AE_AllStages_Action V2.vi"("Velocity"=1.0, "Abort"=w1412, "Positions"=w1415, "Axis"=w1410, "Stage ID"="M686", "Action"=StageStates."MOVE") -> ()  [unwired: 3 in, 3 out]
                    }
                    frame #1 {
                      n639 = call "AE_AllStages_Action V2.vi"("Abort"=w1426, "Axis"=w1424, "Stage ID"="M686", "Action"=StageStates."POSITION") -> ("Position Out"=w1423:dbl[])  [unwired: 5 in, 2 out]
                      n640 = Index Array(array=w1423, index #1=0 ("index"), index #2=1 ("index")) -> (element #1=w1421:dbl, element #2=w1419:dbl)
                      n641 = property on="X" class="DigNum (strict)"("Value"=w1421) -> ()  [unwired: 2 in, 2 out]
                      n642 = property on="Y" class="DigNum (strict)"("Value"=w1419) -> ()  [unwired: 2 in, 2 out]
                    }
                  }
                }
                frame "P841" {
                  n643 = flat-sequence {
                    tunnel: w1433 -> [_]
                    tunnel: w1432 -> [w1438]
                    tunnel: [w1438] -> w1431
                    tunnel: [w1436] -> w1430
                    tunnel: w1429 -> [_]
                    tunnel: w1428 -> [w1434]
                    tunnel: w1431 -> [w1446]
                    tunnel: w1430 -> [w1444]
                    frame #0 {
                      w1436 = bool[] [TRUE] ("Axis")
                      n644 = Build Array(w1434) -> (w1435:dbl[])
                      n645 = call "AE_AllStages_Action V2.vi"("Velocity"=1.0, "Abort"=w1438, "Positions"=w1435, "Axis"=w1436, "Stage ID"="P841", "Action"=StageStates."MOVE") -> ()  [unwired: 3 in, 3 out]
                    }
                    frame #1 {
                      n646 = call "AE_AllStages_Action V2.vi"("Abort"=w1446, "Axis"=w1444, "Stage ID"="P841", "Action"=StageStates."POSITION") -> ("Position Out"=w1443:dbl[])  [unwired: 5 in, 2 out]
                      n647 = Index Array(array=w1443, index #1=0 ("index")) -> (element #1=w1441:dbl)  [unwired: 1 in, 1 out]
                      n648 = property on="Position (µm)" class="DigNum (strict)"("Value"=w1441) -> ()  [unwired: 2 in, 2 out]
                    }
                  }
                }
              }
            }
          }
        }
      }
      event "Exit": Value Change {
        n649 = event-data() -> ("CtlRef"=w1462:refnum<vi>, "NewVal"=w1464:bool)  [unwired: 1 in, 1 out]
        n650 = Release Notifier(notifier=w1453, force destroy? (F)=TRUE) -> ()  [unwired: 1 in, 3 out]
        n651 = property class="Bool"(reference=w1462) -> ("Label.Text"=w1461:string)  [unwired: 1 in, 2 out]
        n652 = call "SLM AE.vi"("Action"=enum16{"READ", "WRITE"}."READ") -> ("SLM Ref Out"=w1451:refnum<vi>)  [unwired: 10 in]
        n653 = call "DM_Ref_AE.vi"("Action"=enum16{"READ", "WRITE"}."READ") -> ("DM Ref Out"=w1449:refnum<vi>)  [unwired: 10 in]
        n654 = call "GateDelay AE.vi"("Action"=enum16{"READ", "WRITE"}."READ") -> ("Gate Delay Ref Out"=w1450:refnum<vi>)  [unwired: 10 in]
        n655 = Enqueue Element(queue=w1463, element=w1461) -> ()  [unwired: 2 in, 3 out]
        n656 = Build Array(w1451, w1449, w1450) -> (w1448:refnum<vi>[])
        n657 = for {
          tunnel: w1448 -> [w1466] mode=indexing
          n658 = Not A Number/Path/Refnum?(number/path/refnum=w1466) -> (NaN/Path/Refnum?=w1465:bool)
          n659 = case shown="False" w1465 {
            tunnel: w1466 -> [w1467 _]
            frame False {
              n660 = To Variant(anything=TRUE) -> (Variant=w1468:variant)
              n661 = invoke class="VI" method="Ctrl Val.Set"(reference=w1467, "Control Name"="Exit", "Value"=w1468) -> (reference out=w1471:refnum<vi>)  [unwired: 2 in, 4 out]
              n662 = Close Reference(reference=w1471) -> ()  [unwired: 1 in, 1 out]
            }
            frame True {
            }
          }
        }
        n663 = Two Button Dialog(message="Record the positions of piezo stages?", 1:"No" ("F button name (\"Cancel\")"), 2:"Yes" ("T button name (\"OK\")")) -> (T button?=w1454:bool)
        n664 = case shown="True" w1454 {
          frame False {
          }
          frame True {
            n665 = Build Array("P612" ("Stage ID"), "M686" ("Stage ID"), "P841" ("Stage ID")) -> (w1476:string[])
            n666 = for {
              tunnel: w1476 -> [w1483] mode=indexing
              tunnel: [w1482] -> w1472 mode=concatenating
              n667 = call "Stage_position_ae.vi"("StageID"=w1483, "Enum"=enum16{"WRITE", "READ"}."READ") -> ("Position Out"=w1482:dbl[])  [unwired: 8 in, 1 out]
            }
            n668 = TDMS Open(10:T24."create or replace" ("operation (0:open)"), 11:path "C:/Users/ED STED/Documents/Test Control Software/Host VIs/Stages/Stage Positions/Stage Positions in Last Experiment.tdms" ("file path")) -> (3:w1478:refnum<k34>)  [unwired: 5 in, 1 out]
            n669 = TDMS Write(0:w1478, 5:"Stage Positions" ("group name in (Untitled)"), 9:w1472) -> (4:w1479:refnum<k34>)  [unwired: 3 in, 3 out]
            n670 = TDMS Close(11:w1479) -> ()  [unwired: 1 in, 2 out]
          }
        }
      }
    }
  }
  n671 = call "Manual Controls Action Engine.vi"("Action"=enum16{"Read", "Write"}."Write", "Manual Controls In"=w25) -> ("Manual Controls Out"=w27:T18)  [unwired: 13 in]
  n672 = call "FPGA-7842R-Control V1.vi"("Action"=FPGA-7842R-Reference."Initialize", "Manual Controls"=w27, "Initialize"=FALSE) -> ("Initalized"=w5:bool)  [unwired: 11 in, 1 out]
  n673 = local write "Upper Shutter"(w13) -> ()
  n674 = local write "Lower Shutter"(w13) -> ()
  n675 = Bundle("Upper Shutter"=w2, "Upper Shutter"=w2) -> (w1:T33)  [unwired: 1 in]
  n676 = call "FPGA-7842R-Control V1.vi"(1:w1, "Action"=FPGA-7842R-Reference."Shutter Control", "Initialize"=w5) -> ("Initalized"=w4:bool)  [unwired: 11 in, 1 out]
  n677 = while {
    shift-right: [w1494] -> _
    shift-left: "Idle" -> [w1495]
    tunnel: w12 -> [w1491]
    shift-right: [w1489] -> _
    shift-left: w4 -> [w1490]
    stop <- w1493 stop-if-true
    n678 = call "Image Aquisition Param Ctrl_AE.vi"("Action"=enum16{"READ", "WRITE"}."READ") -> ("Image Acquisition Parameters Out"=w1488:T15)  [unwired: 10 in]
    n679 = call "Detectors Crl_AE.vi"("Action"=enum16{"READ", "WRITE"}."READ") -> ("Detectors Parameters Out"=w1486:T13)  [unwired: 10 in]
    n680 = case shown="\"Display\"" w1495 {
      selector: w1495 -> [_ _ _ w1527 _ _ _ _ _ _]
      tunnel: ["Exit" w1504 "Idle" ("name (unnamed)") "Arange Displays" ("name (unnamed)") "Start FPGA Acquisition" ("name (unnamed)") "Display" ("name (unnamed)") "Close Images" ("name (unnamed)") "Idle" "Stop Waveforms" ("name (unnamed)") "Start Waveforms" ("name (unnamed)")] -> w1494
      tunnel: [TRUE w1506 w1513 w1535 w1555 w1576 w1617 w1650 w1655 w1661] -> w1493
      tunnel: FALSE -> [_ w1506 w1513 w1535 w1555 w1576 w1617 w1650 w1655 w1661]
      tunnel: w1491 -> [_ w1505 _ _ _ _ _ _ _ _]
      tunnel: w1490 -> [w1500 w1503 w1514 w1533 w1552 w1574 w1615 w1648 w1656 w1662]
      tunnel: [w1499 w1503 w1514 w1533 w1552 w1570 w1615 w1647 w1656 w1662] -> w1489
      tunnel: w1488 -> [_ _ _ w1526 _ w1569 _ _ _ w1659]
      tunnel: w1486 -> [_ _ _ w1525 _ _ _ _ _ w1657]
      frame "Exit" {
        n681 = call "Graph Ref AE.vi"("Action"=enum16{"READ", "WRITE"}."READ") -> ("Graph Ref Out"=w1497:refnum<vi>[])  [unwired: 10 in]
        n682 = call "FPGA-7842R-Control V1.vi"("Action"=FPGA-7842R-Reference."Close FPGA", "Initialize"=w1500) -> ("Initalized"=w1499:bool)  [unwired: 12 in, 1 out]
        n683 = Close Reference(reference=w1497) -> ()  [unwired: 1 in, 1 out]
      }
      frame "Idle", Default {
        n684 = Dequeue Element(queue=w1505, timeout in ms (-1)=-1) -> (element=w1504:string)  [unwired: 1 in, 3 out]
      }
      frame "Close Images" {
        w1509 = u16 0 items=["Read", "Write"] ("Mode")
        w1510 = u16 0 items=["Write", "Read"] ("Mode")
        n685 = call "File Action V1.vi"("Mode"=w1509) -> ("Files Open"=w1508:bool)  [unwired: 12 in, 2 out]
        n686 = call "Image_Actions_V1.vi"("Mode"=w1510, "Action"="Trash Images") -> ()  [unwired: 12 in, 2 out]
        n687 = case shown="True" w1508 {
          frame False {
          }
          frame True {
            w1516 = u16 1 items=["Read", "Write"] ("Mode")
            n688 = call "File Action V1.vi"("Action"="Close Files", "Mode"=w1516) -> ()  [unwired: 11 in, 3 out]
          }
        }
      }
      frame "Capture", "Live" {
        w1531 = u16 0 items=["Write", "Read"] ("Mode")
        n689 = Cluster To Array(cluster=w1525) -> (array=w1523:bool[])
        n690 = Index Array(array=w1523, index=4) -> (element=w1520:bool)
        n691 = Boolean To (0,1)(Boolean=w1523) -> (0, 1=w1524:i16[])
        n692 = Add Array Elements(numeric array=w1524) -> (sum=w1521:i16)
        n693 = To Long Integer(number=w1521) -> (32bit integer=w1518:i32)
        n694 = Unbundle By Name(w1526) -> ("Image Format"=w1528:u16)
        n695 = Select(t=1, s=w1520, f=w1518) -> (s? t:f=w1517:i32)
        n696 = case shown="Default" w1527 {
          tunnel: w1526 -> [_ w1537]
          tunnel: w1517 -> [_ w1536]
          frame Default {
          }
          frame "Capture" {
            w1540 = u16 1 items=["Read", "Write"] ("Mode")
            n697 = call "File Action V1.vi"("Action"="Open Files", "Mode"=w1540, "Image Acquisition Parameters"=w1537, "File Path IN"="Save File Path", "Number of Channels"=w1536) -> ("File Path OUT"=w1538:path)  [unwired: 8 in, 2 out]
            n698 = local write "Save File Path"(w1538) -> ()
          }
        }
        n699 = To Long Integer(number=w1528) -> (32bit integer=w1530:i32)
        n700 = Bundle(w1530, w1530) -> (w1529:cluster{i32, i32})  [unwired: 1 in]
        n701 = call "Image_Actions_V1.vi"("Image Size (Pixels)"=w1529, "Mode"=w1531, "Number of Channels"=w1517, "Action"="Create Images") -> ()  [unwired: 10 in, 2 out]
      }
      frame "Arange Displays" {
        w1550 = u16 1 items=["Write", "Read"] ("Mode")
        w1553 = u16 1 items=["Read", "Write"] ("Action")
        n702 = call "Graph Ref AE.vi"("Action"=enum16{"READ", "WRITE"}."READ") -> ("Graph Ref Out"=w1545:refnum<vi>[])  [unwired: 10 in]
        n703 = call "Image_Actions_V1.vi"("Mode"=w1550) -> ("Image REFs OUT"=w1551:T35[])  [unwired: 13 in, 1 out]
        n704 = Array Size(array=w1551) -> (size(s)=w1549:i32)
        n705 = call "Arange_Displays_V2.vi"("Display References"=w1545, "Action"=w1553, "Number of Channels"=w1549, "Aspect Ratio (h/w)"=1.0) -> ("Number of Channels OUT"=w1546:i32)  [unwired: 11 in]
        n706 = for {
          N: w1546 -> [_]
          tunnel: w1545 -> [w1557] mode=indexing
          tunnel: [w1560] -> w1547 mode=indexing
          i -> [w1558]
          n707 = property class="IntGraph (strict)"(reference=w1557) -> ("Label.Text"=w1562:string)  [unwired: 1 in, 2 out]
          n708 = Equal To 0?(x=w1558) -> (x = 0?=w1559:bool)
          n709 = case shown="True" w1559 {
            tunnel: w1557 -> [_ w1563]
            frame False {
            }
            frame True {
              n710 = property class="IntGraph (strict)"(reference=w1563, "ZScale.Visible"=TRUE ("Z Scale.Visible"), "ZScale.Position"=T20 {"Left"=2308, "Top"=-340} ("Z Scale.Position")) -> ()  [unwired: 1 in, 2 out]
            }
          }
          n711 = To Unsigned Word Integer(number=w1558) -> (unsigned 16bit integer=w1561:u16)
          n712 = Bundle("Label.Text"=w1562, w1561) -> (w1560:cluster{"Label.Text":string, u16})  [unwired: 1 in]
        }
        n713 = property on="Active Channel" class="Ring (strict)"("StringsAndValues[]"=w1547) -> (error out=w1544:errorcluster)  [unwired: 2 in, 1 out]
        n714 = local write "Graph Mode"(T34."GetIntensity" ("Graph Mode")) -> ()
        n715 = property on="Active Channel" class="Ring (strict)"(error in=w1544, "Value"=u16 0) -> ()  [unwired: 1 in, 2 out]
      }
      frame "Start Waveforms" {
        n716 = call "Initialize Waveforms V4.vi"("Image Acquisition Parameters"=w1569) -> ("Waveform Data to FPGA"=w1575:T36)  [unwired: 14 in]
        n717 = Unbundle By Name(w1569) -> ("Scan Type"=w1568:enum16{"Sample Scanning", "Beam Scanning"})
        n718 = call "FPGA-7842R-Control V1.vi"("Waveform Data"=w1575, "Action"=FPGA-7842R-Reference."Start Waveforms", "Image Acquisition Parameters"=w1569, "Initialize"=w1574) -> ("Initalized"=w1571:bool)  [unwired: 10 in, 1 out]
        n719 = Equal?(x=w1568, y=enum16{"Sample Scanning", "Beam Scanning"}."Sample Scanning" ("Scan Type")) -> (x = y?=w1566:bool)
        n720 = case shown="False" w1566 {
          tunnel: w1571 -> [w1577 w1582]
          tunnel: [w1577 w1581] -> w1570
          frame False {
          }
          frame True {
            n721 = call "Scan Parameters Action Engine.vi"("Action"=enum16{"Read", "Write"}."Read") -> ("Scan Parameters OUT"=w1579:T17)  [unwired: 14 in]
            n722 = Unbundle By Name(w1579) -> ("Unused_Axis_I16"=w1578:i16)
            n723 = call "FPGA-7842R-Control V1.vi"("Action"=FPGA-7842R-Reference."Unused Axis I16", "Initialize"=w1582, "Unused Axis Offset (I16)"=w1578) -> ("Initalized"=w1581:bool)  [unwired: 11 in, 1 out]
          }
        }
      }
      frame "Display" {
        w1610 = u16 1 items=["Write", "Read"] ("Mode")
        n724 = call "Image_Actions_V1.vi"("Mode"=w1610) -> ("Image REFs OUT"=w1612:T35[])  [unwired: 13 in, 1 out]
        n725 = Array Size(array=w1612) -> (size(s)=w1608:i32)
        n726 = Decrement(x=w1608) -> (x-1=w1607:i32)
        n727 = for {
          N: 6 -> [_]
          tunnel: w1607 -> [w1645]
          tunnel: [w1643] -> w1611 mode=indexing
          i -> [w1644]
          n728 = Greater Or Equal?(x=w1645, y=w1644) -> (x >= y?=w1643:bool)
        }
        n729 = Obtain Notifier(name (unnamed)="Running", notification data type=FALSE) -> (notifier out=w1584:refnum<notifier>)  [unwired: 2 in, 2 out]
        n730 = Index Array(array=w1611, index #1=1 ("index"), index #2=2 ("index"), index #3=3 ("index"), index #4=4 ("index"), index #5=5 ("index")) -> (element #1=w1596:bool, element #2=w1595:bool, element #3=w1594:bool, element #4=w1593:bool, element #5=w1592:bool)
        n731 = Index Array(array=w1612, index #1=0 ("index"), index #2=1 ("index"), index #3=2 ("index"), index #4=3 ("index"), index #5=4 ("index"), index #6=5 ("index")) -> (element #1=w1591:T35, element #2=w1590:T35, element #3=w1589:T35, element #4=w1588:T35, element #5=w1587:T35, element #6=w1586:T35)
        n732 = while {
          tunnel: w1596 -> [w1632]
          tunnel: w1595 -> [w1631]
          tunnel: w1594 -> [w1627]
          tunnel: w1593 -> [w1624]
          tunnel: w1592 -> [w1623]
          tunnel: w1591 -> [w1630]
          tunnel: w1590 -> [w1629]
          tunnel: w1589 -> [w1628]
          tunnel: w1588 -> [w1626]
          tunnel: w1587 -> [w1622]
          tunnel: w1586 -> [w1625]
          tunnel: w1584 -> [w1618]
          stop <- w1619 stop-if-true
          n733 = Get Notifier Status(notifier=w1618) -> (current notification=w1619:bool)  [unwired: 1 in, 4 out]
          n734 = case shown="False" w1632 {
            tunnel: w1629 -> [_ w1642]
            frame False {
            }
            frame True {
              n735 = call "IMAQ ImageToArray"("Image"=w1642) -> ("Image Pixels (Float)"=→"Channel 2":sgl[][])  [unwired: 3 in, 4 out]
            }
          }
          n736 = case shown="False" w1631 {
            tunnel: w1628 -> [_ w1640]
            frame False {
            }
            frame True {
              n737 = call "IMAQ ImageToArray"("Image"=w1640) -> ("Image Pixels (Float)"=→"Channel 3":sgl[][])  [unwired: 3 in, 4 out]
            }
          }
          n738 = call "IMAQ ImageToArray"("Image"=w1630) -> ("Image Pixels (Float)"=→"Channel 1":sgl[][])  [unwired: 3 in, 4 out]
          n739 = case shown="False" w1627 {
            tunnel: w1626 -> [_ w1638]
            frame False {
            }
            frame True {
              n740 = call "IMAQ ImageToArray"("Image"=w1638) -> ("Image Pixels (Float)"=→"Channel 4":sgl[][])  [unwired: 3 in, 4 out]
            }
          }
          n741 = case shown="False" w1624 {
            tunnel: w1622 -> [_ w1636]
            frame False {
            }
            frame True {
              n742 = call "IMAQ ImageToArray"("Image"=w1636) -> ("Image Pixels (Float)"=→"Channel 5":sgl[][])  [unwired: 3 in, 4 out]
            }
          }
          n743 = case shown="False" w1623 {
            tunnel: w1625 -> [_ w1634]
            frame False {
            }
            frame True {
              n744 = call "IMAQ ImageToArray"("Image"=w1634) -> ("Image Pixels (Float)"=→"Channel 6":sgl[][])  [unwired: 3 in, 4 out]
            }
          }
          n745 = Wait (ms)(milliseconds to wait=u32 100) -> ()  [unwired: 1 out]
        }
      }
      frame "Stop Waveforms" {
        n746 = call "FPGA-7842R-Control V1.vi"("Action"=FPGA-7842R-Reference."Stop Waveforms", "Initialize"=w1648) -> ("Initalized"=w1647:bool)  [unwired: 12 in, 1 out]
      }
      frame "Stop Acquisition" {
        n747 = call "FPGA-7842R-Control V1.vi"("Action"=FPGA-7842R-Reference."Laser Control", "Laser Controls"=T14 {"STED Power (V)"=0.0, "STED"=FALSE, "640 nm"=FALSE, "590 nm"=FALSE, "485 nm"=FALSE, "Manual Control"=FALSE} ("Laser Controls 2"), "Initialize"=TRUE) -> ()  [unwired: 11 in, 2 out]
      }
      frame "Start FPGA Acquisition" {
        n748 = Unbundle By Name(w1659) -> ("Scan Mode"=w1658:enum16{"XY", "XZ", "YZ", "XYZ"})
        n749 = case shown="\"XZ\", Default" w1658 {
          tunnel: w1659 -> [_ w1669]
          tunnel: w1657 -> [_ w1670]
          frame "YZ" {
            n750 = vi-ref "FPGA Sample Scanning V1.vi"() -> (w1665:refnum<vi>)
            n751 = property class="VI Interface Type 3"(reference=w1665) -> ("Path"=w1663:path)  [unwired: 1 in, 2 out]
            n752 = Open VI Reference(type specifier VI Refnum (for type only)=w1665, vi path=w1663, options=128) -> (vi reference=w1666:refnum<vi>)  [unwired: 3 in, 1 out]
            n753 = call-by-ref "Start Asynchronous Call"(reference=w1666) -> (reference out=w1667:refnum<vi>)  [unwired: 4 in, 1 out]
            n754 = Close Reference(reference=w1667) -> ()  [unwired: 1 in, 1 out]
          }
          frame "XZ", Default {
            n755 = vi-ref "FPGA Beam Scanning V1.vi"() -> (w1668:refnum<vi>)
            n756 = property class="VI Interface Type 4"(reference=w1668) -> ("Path"=w1672:path)  [unwired: 1 in, 2 out]
            n757 = Open VI Reference(type specifier VI Refnum (for type only)=w1668, vi path=w1672, options=128) -> (vi reference=w1671:refnum<vi>)  [unwired: 3 in, 1 out]
            n758 = call-by-ref "Start Asynchronous Call"(reference=w1671, "Detectors"=w1670, "Image Acquisition Parameters"=w1669) -> (reference out=w1674:refnum<vi>)  [unwired: 2 in, 1 out]
            n759 = Close Reference(reference=w1674) -> ()  [unwired: 1 in, 1 out]
          }
        }
      }
    }
  }
